vi "Text control 2 v4.9_pump-specific.vi"() -> ()   [LabVIEW 2016]
panel:
  in  "Tab Control":enum32{"Main", "Other parameters"}(tab)
  out "Line running":i32
  out "Total lines":i32
  out "Path":path=path "C:/users/rlp38/09Apr2009LTtesting/test2.txt"
  out "I vs Vg":cluster{"Y data in":dbl[], "X data in":dbl[]}[](graph)
  out "Is":dbl format="%.2e"
  out "Id":dbl format="%.2e"
  out "Ig":dbl format="%.2e"
  out "Id max vs time":cluster{"Y data in":dbl[], "X data in":dbl[]}[](graph)
  out "Id min vs time":cluster{"Y data in":dbl[], "X data in":dbl[]}[](graph)
  out "I vs Vd":cluster{"Y data in":dbl[], "X data in":dbl[]}[](graph)
  in  "Program":string="#-------------------------------------------------------\n# Liquid cycling script\n# Version 0.1\n# Author: Dimitrios Simatos\n# Last updated: 2017-10-12\n#-------------------------------------------------------\n# Things to do before running the script:\n# Set time units to minutes.\n# Set filenames.\n# Replace the tubing, if necessary.\n#-------------------------------------------------------\n# Port connections\n# Port 1: Waste\n# Port 2: Device\n# Port 3: Ultrapure water\n# Port 4: Nothing\n# Port 5: Nothing\n# Port 6: Nothing\n#-------------------------------------------------------\n# Execution time: 4 x 30 = 120 minutes = 2 hours\n# This script is designed to perform a cycling experiment between two liquids.\n# There are 4 pumping cycles, each one followed by 30 minutes of measurements.\n# All cycles pump ultrapure water (port 3).\n# Flow V = 20 pulses/second (400 ul/min)\n#-------------------------------------------------------\n# Cycle 1\npump /1ZR #initialize pump\npump /1Q #query pump\ntransfer d 1 -1 -0.1 -1 -1 0\npump /1? #report absolute plunger position\npump /1?6 #report valve position\nwait-min 1 #wait 1 minute\ntransfer d 1 -1 -0.1 -1 -1 0\npump /1N0R #set step resolution: 0.01 mm\npump /1Q #query pump\npump /1? #report absolute plunger position (the plunger should be at 0)\npump /1?6 #report valve position\nwait 1000 #wait 1 second\npump /1V300R #choose speed: 300 steps/s\npump /1Q #query pump\nwait 1000 #wait 1 second\npump /1O3R #go to port 3, counterclockwise rotation\npump /1Q #query pump\nwait 1000 #wait 1 second\npump /1A2400R #go to absolute position 2400\nwait 20000 #wait 20 seconds\npump /1V20R #set speed to 20 steps/s\npump /1Q #query pump\nwait 10000 # wait 10 seconds\ntransfer d 1 -1 -0.1 -1 -1 0\npump /1? #report absolute plunger position (the plunger should have finished moving)\npump /1?6 #report valve position\npump /1O2R #switch to port 2, counterclockwise rotation\npump /1Q #query pump\nwait 200 #wait 200 milliseconds\npump /1A0R #go to absolute position 0 (= empty syringe)\npump /1Q #query pump\npump /1? #report absolute plunger position (the plunger should be moving to 0)\npump /1?6 #report valve position\ntransfer d 1 -1 -0.1 -1 -1 0\nwait-min 1\npump /1Q #query pump\npump /1? #report absolute plunger position (the plunger should be moving to 0)\npump /1?6 #report valve position\ntransfer d 1 -1 -0.1 -1 -1 0\nwait-min 1\npump /1Q #query pump\npump /1? #report absolute plunger position\npump /1?6 #report valve position\ntransfer d 1 -1 -0.1 -1 -1 0\nwait-min 1\npump /1Q #query pump\npump /1? #report absolute plunger position\npump /1?6 #report valve position\ntransfer d 1 -1 -0.1 -1 -1 0\nwait-min 1\npump /1Q #query pump\npump /1? #report absolute plunger position\npump /1?6 #report valve position\ntransfer d 1 -1 -0.1 -1 -1 0\nwait-min 1\npump /1Q #query pump\npump /1? #report absolute plunger position\npump /1?6 #report valve position\ntransfer d 1 -1 -0.1 -1 -1 0\nwait-min 1\npump /1Q #query pump\npump /1? #report absolute plunger position\npump /1?6 #report valve position\ntransfer d 1 -1 -0.1 -1 -1 0\nwait-min 1\npump /1Q #query pump\npump /1? #report absolute plunger position\npump /1?6 #report valve position\ntransfer d 1 -1 -0.1 -1 -1 0\nwait-min 1\npump /1Q #query pump\npump /1? #report absolute plunger position\npump /1?6 #report valve position\ntransfer d 1 -1 -0.1 -1 -1 0\nwait-min 1\npump /1Q #query pump\npump /1? #report absolute plunger position\npump /1?6 #report valve position\ntransfer d 1 -1 -0.1 -1 -1 0\nwait-min 1\npump /1Q #query pump\npump /1? #report absolute plunger position\npump /1?6 #report valve position\ntransfer d 1 -1 -0.1 -1 -1 0\nwait-min 1\npump /1Q #query pump\npump /1? #report absolute plunger position\npump /1?6 #report valve position\ntransfer d 1 -1 -0.1 -1 -1 0\nwait-min 1\npump /1Q #query pump\npump /1? #report absolute plunger position\npump /1?6 #report valve position\ntransfer d 1 -1 -0.1 -1 -1 0\nwait-min 1\npump /1Q #query pump\npump /1? #report absolute plunger position\npump /1?6 #report valve position\ntransfer d 1 -1 -0.1 -1 -1 0\nwait-min 1\npump /1Q #query pump\npump /1? #report absolute plunger position\npump /1?6 #report valve position\ntransfer d 1 -1 -0.1 -1 -1 0\nwait-min 1\npump /1Q #query pump\npump /1? #report absolute plunger position\npump /1?6 #report valve position\ntransfer d 1 -1 -0.1 -1 -1 0\nwait-min 1\npump /1Q #query pump\npump /1? #report absolute plunger position\npump /1?6 #report valve position\ntransfer d 1 -1 -0.1 -1 -1 0\nwait-min 1\npump /1Q #query pump\npump /1? #report absolute plunger position\npump /1?6 #report valve position\ntransfer d 1 -1 -0.1 -1 -1 0\nwait-min 1\npump /1Q #query pump\npump /1? #report absolute plunger position\npump /1?6 #report valve position\ntransfer d 1 -1 -0.1 -1 -1 0\nwait-min 1\npump /1Q #query pump\npump /1? #report absolute plunger position\npump /1?6 #report valve position\ntransfer d 1 -1 -0.1 -1 -1 0\nwait-min 1\npump /1Q #query pump\npump /1? #report absolute plunger position\npump /1?6 #report valve position\ntransfer d 1 -1 -0.1 -1 -1 0\nwait-min 1\npump /1Q #query pump\npump /1? #report absolute plunger position\npump /1?6 #report valve position\ntransfer d 1 -1 -0.1 -1 -1 0\nwait-min 1\npump /1Q #query pump\npump /1? #report absolute plunger position\npump /1?6 #report valve position\ntransfer d 1 -1 -0.1 -1 -1 0\nwait-min 1\npump /1Q #query pump\npump /1? #report absolute plunger position\npump /1?6 #report valve position\ntransfer d 1 -1 -0.1 -1 -1 0\nwait-min 1\npump /1Q #query pump\npump /1? #report absolute plunger position\npump /1?6 #report valve position\ntransfer d 1 -1 -0.1 -1 -1 0\nwait-min 1\n#-------------------------------------------------------\n# Cycle 2\npump /1ZR #initialize pump\npump /1Q #query pump\ntransfer d 1 -1 -0.1 -1 -1 0\npump /1? #report absolute plunger position\npump /1?6 #report valve position\nwait-min 1 #wait 1 minute\ntransfer d 1 -1 -0.1 -1 -1 0\npump /1N0R #set step resolution: 0.01 mm\npump /1Q #query pump\npump /1? #report absolute plunger position (the plunger should be at 0)\npump /1?6 #report valve position\nwait 1000 #wait 1 second\npump /1V300R #choose speed: 300 steps/s\npump /1Q #query pump\nwait 1000 #wait 1 second\npump /1O3R #go to port 3, counterclockwise rotation\npump /1Q #query pump\nwait 1000 #wait 1 second\npump /1A2400R #go to absolute position 2400\nwait 20000 #wait 20 seconds\ntransfer d 1 -1 -0.1 -1 -1 0\npump /1V20R #set speed to 20 steps/s\npump /1Q #query pump\nwait 10000 # wait 10 seconds\npump /1? #report absolute plunger position (the plunger should have finished moving)\npump /1?6 #report valve position\npump /1O2R #switch to port 2, counterclockwise rotation\npump /1Q #query pump\nwait 200 #wait 200 milliseconds\npump /1A0R #go to absolute position 0 (= empty syringe)\npump /1Q #query pump\npump /1? #report absolute plunger position (the plunger should be moving to 0)\npump /1?6 #report valve position\ntransfer d 1 -1 -0.1 -1 -1 0\nwait-min 1\npump /1Q #query pump\npump /1? #report absolute plunger position (the plunger should be moving to 0)\npump /1?6 #report valve position\ntransfer d 1 -1 -0.1 -1 -1 0\nwait-min 1\npump /1Q #query pump\npump /1? #report absolute plunger position\npump /1?6 #report valve position\ntransfer d 1 -1 -0.1 -1 -1 0\nwait-min 1\npump /1Q #query pump\npump /1? #report absolute plunger position\npump /1?6 #report valve position\ntransfer d 1 -1 -0.1 -1 -1 0\nwait-min 1\npump /1Q #query pump\npump /1? #report absolute plunger position\npump /1?6 #report valve position\ntransfer d 1 -1 -0.1 -1 -1 0\nwait-min 1\npump /1Q #query pump\npump /1? #report absolute plunger position\npump /1?6 #report valve position\ntransfer d 1 -1 -0.1 -1 -1 0\nwait-min 1\npump /1Q #query pump\npump /1? #report absolute plunger position\npump /1?6 #report valve position\ntransfer d 1 -1 -0.1 -1 -1 0\nwait-min 1\npump /1Q #query pump\npump /1? #report absolute plunger position\npump /1?6 #report valve position\ntransfer d 1 -1 -0.1 -1 -1 0\nwait-min 1\npump /1Q #query pump\npump /1? #report absolute plunger position\npump /1?6 #report valve position\ntransfer d 1 -1 -0.1 -1 -1 0\nwait-min 1\npump /1Q #query pump\npump /1? #report absolute plunger position\npump /1?6 #report valve position\ntransfer d 1 -1 -0.1 -1 -1 0\nwait-min 1\npump /1Q #query pump\npump /1? #report absolute plunger position\npump /1?6 #report valve position\ntransfer d 1 -1 -0.1 -1 -1 0\nwait-min 1\npump /1Q #query pump\npump /1? #report absolute plunger position\npump /1?6 #report valve position\ntransfer d 1 -1 -0.1 -1 -1 0\nwait-min 1\npump /1Q #query pump\npump /1? #report absolute plunger position\npump /1?6 #report valve position\ntransfer d 1 -1 -0.1 -1 -1 0\nwait-min 1\npump /1Q #query pump\npump /1? #report absolute plunger position\npump /1?6 #report valve position\ntransfer d 1 -1 -0.1 -1 -1 0\nwait-min 1\npump /1Q #query pump\npump /1? #report absolute plunger position\npump /1?6 #report valve position\ntransfer d 1 -1 -0.1 -1 -1 0\nwait-min 1\npump /1Q #query pump\npump /1? #report absolute plunger position\npump /1?6 #report valve position\ntransfer d 1 -1 -0.1 -1 -1 0\nwait-min 1\npump /1Q #query pump\npump /1? #report absolute plunger position\npump /1?6 #report valve position\ntransfer d 1 -1 -0.1 -1 -1 0\nwait-min 1\npump /1Q #query pump\npump /1? #report absolute plunger position\npump /1?6 #report valve position\ntransfer d 1 -1 -0.1 -1 -1 0\nwait-min 1\npump /1Q #query pump\npump /1? #report absolute plunger position\npump /1?6 #report valve position\ntransfer d 1 -1 -0.1 -1 -1 0\nwait-min 1\npump /1Q #query pump\npump /1? #report absolute plunger position\npump /1?6 #report valve position\ntransfer d 1 -1 -0.1 -1 -1 0\nwait-min 1\npump /1Q #query pump\npump /1? #report absolute plunger position\npump /1?6 #report valve position\ntransfer d 1 -1 -0.1 -1 -1 0\nwait-min 1\npump /1Q #query pump\npump /1? #report absolute plunger position\npump /1?6 #report valve position\ntransfer d 1 -1 -0.1 -1 -1 0\nwait-min 1\npump /1Q #query pump\npump /1? #report absolute plunger position\npump /1?6 #report valve position\ntransfer d 1 -1 -0.1 -1 -1 0\nwait-min 1\npump /1Q #query pump\npump /1? #report absolute plunger position\npump /1?6 #report valve position\ntransfer d 1 -1 -0.1 -1 -1 0\nwait-min 1\npump /1Q #query pump\npump /1? #report absolute plunger position\npump /1?6 #report valve position\ntransfer d 1 -1 -0.1 -1 -1 0\nwait-min 1\n#-------------------------------------------------------\n# Cycle 3\npump /1ZR #initialize pump\npump /1Q #query pump\ntransfer d 1 -1 -0.1 -1 -1 0\npump /1? #report absolute plunger position\npump /1?6 #report valve position\nwait-min 1 #wait 1 minute\ntransfer d 1 -1 -0.1 -1 -1 0\npump /1N0R #set step resolution: 0.01 mm\npump /1Q #query pump\npump /1? #report absolute plunger position (the plunger should be at 0)\npump /1?6 #report valve position\nwait 1000 #wait 1 second\npump /1V300R #choose speed: 300 steps/s\npump /1Q #query pump\nwait 1000 #wait 1 second\npump /1O3R #go to port 3, counterclockwise rotation\npump /1Q #query pump\nwait 1000 #wait 1 second\npump /1A2400R #go to absolute position 2400\nwait 20000 #wait 20 seconds\ntransfer d 1 -1 -0.1 -1 -1 0\npump /1V20R #set speed to 20 steps/s\npump /1Q #query pump\nwait 10000 # wait 10 seconds\npump /1? #report absolute plunger position (the plunger should have finished moving)\npump /1?6 #report valve position\npump /1O2R #switch to port 2, counterclockwise rotation\npump /1Q #query pump\nwait 200 #wait 200 milliseconds\npump /1A0R #go to absolute position 0 (= empty syringe)\npump /1Q #query pump\npump /1? #report absolute plunger position (the plunger should be moving to 0)\npump /1?6 #report valve position\ntransfer d 1 -1 -0.1 -1 -1 0\nwait-min 1\npump /1Q #query pump\npump /1? #report absolute plunger position (the plunger should be moving to 0)\npump /1?6 #report valve position\ntransfer d 1 -1 -0.1 -1 -1 0\nwait-min 1\npump /1Q #query pump\npump /1? #report absolute plunger position\npump /1?6 #report valve position\ntransfer d 1 -1 -0.1 -1 -1 0\nwait-min 1\npump /1Q #query pump\npump /1? #report absolute plunger position\npump /1?6 #report valve position\ntransfer d 1 -1 -0.1 -1 -1 0\nwait-min 1\npump /1Q #query pump\npump /1? #report absolute plunger position\npump /1?6 #report valve position\ntransfer d 1 -1 -0.1 -1 -1 0\nwait-min 1\npump /1Q #query pump\npump /1? #report absolute plunger position\npump /1?6 #report valve position\ntransfer d 1 -1 -0.1 -1 -1 0\nwait-min 1\npump /1Q #query pump\npump /1? #report absolute plunger position\npump /1?6 #report valve position\ntransfer d 1 -1 -0.1 -1 -1 0\nwait-min 1\npump /1Q #query pump\npump /1? #report absolute plunger position\npump /1?6 #report valve position\ntransfer d 1 -1 -0.1 -1 -1 0\nwait-min 1\npump /1Q #query pump\npump /1? #report absolute plunger position\npump /1?6 #report valve position\ntransfer d 1 -1 -0.1 -1 -1 0\nwait-min 1\npump /1Q #query pump\npump /1? #report absolute plunger position\npump /1?6 #report valve position\ntransfer d 1 -1 -0.1 -1 -1 0\nwait-min 1\npump /1Q #query pump\npump /1? #report absolute plunger position\npump /1?6 #report valve position\ntransfer d 1 -1 -0.1 -1 -1 0\nwait-min 1\npump /1Q #query pump\npump /1? #report absolute plunger position\npump /1?6 #report valve position\ntransfer d 1 -1 -0.1 -1 -1 0\nwait-min 1\npump /1Q #query pump\npump /1? #report absolute plunger position\npump /1?6 #report valve position\ntransfer d 1 -1 -0.1 -1 -1 0\nwait-min 1\npump /1Q #query pump\npump /1? #report absolute plunger position\npump /1?6 #report valve position\ntransfer d 1 -1 -0.1 -1 -1 0\nwait-min 1\npump /1Q #query pump\npump /1? #report absolute plunger position\npump /1?6 #report valve position\ntransfer d 1 -1 -0.1 -1 -1 0\nwait-min 1\npump /1Q #query pump\npump /1? #report absolute plunger position\npump /1?6 #report valve position\ntransfer d 1 -1 -0.1 -1 -1 0\nwait-min 1\npump /1Q #query pump\npump /1? #report absolute plunger position\npump /1?6 #report valve position\ntransfer d 1 -1 -0.1 -1 -1 0\nwait-min 1\npump /1Q #query pump\npump /1? #report absolute plunger position\npump /1?6 #report valve position\ntransfer d 1 -1 -0.1 -1 -1 0\nwait-min 1\npump /1Q #query pump\npump /1? #report absolute plunger position\npump /1?6 #report valve position\ntransfer d 1 -1 -0.1 -1 -1 0\nwait-min 1\npump /1Q #query pump\npump /1? #report absolute plunger position\npump /1?6 #report valve position\ntransfer d 1 -1 -0.1 -1 -1 0\nwait-min 1\npump /1Q #query pump\npump /1? #report absolute plunger position\npump /1?6 #report valve position\ntransfer d 1 -1 -0.1 -1 -1 0\nwait-min 1\npump /1Q #query pump\npump /1? #report absolute plunger position\npump /1?6 #report valve position\ntransfer d 1 -1 -0.1 -1 -1 0\nwait-min 1\npump /1Q #query pump\npump /1? #report absolute plunger position\npump /1?6 #report valve position\ntransfer d 1 -1 -0.1 -1 -1 0\nwait-min 1\npump /1Q #query pump\npump /1? #report absolute plunger position\npump /1?6 #report valve position\ntransfer d 1 -1 -0.1 -1 -1 0\nwait-min 1\npump /1Q #query pump\npump /1? #report absolute plunger position\npump /1?6 #report valve position\ntransfer d 1 -1 -0.1 -1 -1 0\nwait-min 1\n#-------------------------------------------------------\n# Cycle 4\npump /1ZR #initialize pump\npump /1Q #query pump\ntransfer d 1 -1 -0.1 -1 -1 0\npump /1? #report absolute plunger position\npump /1?6 #report valve position\nwait-min 1 #wait 1 minute\ntransfer d 1 -1 -0.1 -1 -1 0\npump /1N0R #set step resolution: 0.01 mm\npump /1Q #query pump\npump /1? #report absolute plunger position (the plunger should be at 0)\npump /1?6 #report valve position\nwait 1000 #wait 1 second\npump /1V300R #choose speed: 300 steps/s\npump /1Q #query pump\nwait 1000 #wait 1 second\npump /1O3R #go to port 3, counterclockwise rotation\npump /1Q #query pump\nwait 1000 #wait 1 second\npump /1A2400R #go to absolute position 2400\nwait 20000 #wait 20 seconds\ntransfer d 1 -1 -0.1 -1 -1 0\npump /1V20R #set speed to 20 steps/s\npump /1Q #query pump\nwait 10000 # wait 10 seconds\npump /1? #report absolute plunger position (the plunger should have finished moving)\npump /1?6 #report valve position\npump /1O2R #switch to port 2, counterclockwise rotation\npump /1Q #query pump\nwait 200 #wait 200 milliseconds\npump /1A0R #go to absolute position 0 (= empty syringe)\npump /1Q #query pump\npump /1? #report absolute plunger position (the plunger should be moving to 0)\npump /1?6 #report valve position\ntransfer d 1 -1 -0.1 -1 -1 0\nwait-min 1\npump /1Q #query pump\npump /1? #report absolute plunger position (the plunger should be moving to 0)\npump /1?6 #report valve position\ntransfer d 1 -1 -0.1 -1 -1 0\nwait-min 1\npump /1Q #query pump\npump /1? #report absolute plunger position\npump /1?6 #report valve position\ntransfer d 1 -1 -0.1 -1 -1 0\nwait-min 1\npump /1Q #query pump\npump /1? #report absolute plunger position\npump /1?6 #report valve position\ntransfer d 1 -1 -0.1 -1 -1 0\nwait-min 1\npump /1Q #query pump\npump /1? #report absolute plunger position\npump /1?6 #report valve position\ntransfer d 1 -1 -0.1 -1 -1 0\nwait-min 1\npump /1Q #query pump\npump /1? #report absolute plunger position\npump /1?6 #report valve position\ntransfer d 1 -1 -0.1 -1 -1 0\nwait-min 1\npump /1Q #query pump\npump /1? #report absolute plunger position\npump /1?6 #report valve position\ntransfer d 1 -1 -0.1 -1 -1 0\nwait-min 1\npump /1Q #query pump\npump /1? #report absolute plunger position\npump /1?6 #report valve position\ntransfer d 1 -1 -0.1 -1 -1 0\nwait-min 1\npump /1Q #query pump\npump /1? #report absolute plunger position\npump /1?6 #report valve position\ntransfer d 1 -1 -0.1 -1 -1 0\nwait-min 1\npump /1Q #query pump\npump /1? #report absolute plunger position\npump /1?6 #report valve position\ntransfer d 1 -1 -0.1 -1 -1 0\nwait-min 1\npump /1Q #query pump\npump /1? #report absolute plunger position\npump /1?6 #report valve position\ntransfer d 1 -1 -0.1 -1 -1 0\nwait-min 1\npump /1Q #query pump\npump /1? #report absolute plunger position\npump /1?6 #report valve position\ntransfer d 1 -1 -0.1 -1 -1 0\nwait-min 1\npump /1Q #query pump\npump /1? #report absolute plunger position\npump /1?6 #report valve position\ntransfer d 1 -1 -0.1 -1 -1 0\nwait-min 1\npump /1Q #query pump\npump /1? #report absolute plunger position\npump /1?6 #report valve position\ntransfer d 1 -1 -0.1 -1 -1 0\nwait-min 1\npump /1Q #query pump\npump /1? #report absolute plunger position\npump /1?6 #report valve position\ntransfer d 1 -1 -0.1 -1 -1 0\nwait-min 1\npump /1Q #query pump\npump /1? #report absolute plunger position\npump /1?6 #report valve position\ntransfer d 1 -1 -0.1 -1 -1 0\nwait-min 1\npump /1Q #query pump\npump /1? #report absolute plunger position\npump /1?6 #report valve position\ntransfer d 1 -1 -0.1 -1 -1 0\nwait-min 1\npump /1Q #query pump\npump /1? #report absolute plunger position\npump /1?6 #report valve position\ntransfer d 1 -1 -0.1 -1 -1 0\nwait-min 1\npump /1Q #query pump\npump /1? #report absolute plunger position\npump /1?6 #report valve position\ntransfer d 1 -1 -0.1 -1 -1 0\nwait-min 1\npump /1Q #query pump\npump /1? #report absolute plunger position\npump /1?6 #report valve position\ntransfer d 1 -1 -0.1 -1 -1 0\nwait-min 1\npump /1Q #query pump\npump /1? #report absolute plunger position\npump /1?6 #report valve position\ntransfer d 1 -1 -0.1 -1 -1 0\nwait-min 1\npump /1Q #query pump\npump /1? #report absolute plunger position\npump /1?6 #report valve position\ntransfer d 1 -1 -0.1 -1 -1 0\nwait-min 1\npump /1Q #query pump\npump /1? #report absolute plunger position\npump /1?6 #report valve position\ntransfer d 1 -1 -0.1 -1 -1 0\nwait-min 1\npump /1Q #query pump\npump /1? #report absolute plunger position\npump /1?6 #report valve position\ntransfer d 1 -1 -0.1 -1 -1 0\nwait-min 1\npump /1Q #query pump\npump /1? #report absolute plunger position\npump /1?6 #report valve position\ntransfer d 1 -1 -0.1 -1 -1 0\nwait-min 1\n#-------------------------------------------------------"
  out "Command running:":string="#output s 0 0 0 -0.008 0.008 0.002"
  out "Serial port data":string
  out "Elapsed Time":dbl caption="Elapsed Time (s)"
  in  "Units":u16(ring)=1 items=["Seconds", "Minutes", "Hours"]
  in  "Time Offset":dbl caption="Set Start Time (s)"
  in  "Reset":bool
  in  "Auto Reset":bool
  in  "integration time":u32(slide) max=2 step=1 scale=0.0..2.0
  in  "Interrupt run":bool
  out "Absolute plunger position vs time":cluster{"Y data in":dbl[], "X data in":dbl[]}[](graph)
  out "Valve position vs time":cluster{"Y data in":dbl[], "X data in":dbl[]}[](graph)
  in  "Halt pump":bool
  in  "Hard stop pump":bool
  in  "Gate Range\nmode":u16(ring) items=["Auto", "Limited", "Fixed"]
  in  "Gate Range":u8(slide)=6 max=11 scale=0.0..11.0
  in  "Source/Drain\nRange mode":u16(ring) items=["Auto", "Limited", "Fixed"]
  in  "Source/Drain Range":u8(slide)=6 max=11 scale=0.0..11.0
  in  "Panel Controls":T1={"Emergency Stop"=refnum, "TransGraph Max"=1e-05, "Text/Graph (text=false)"=TRUE} {"TransGraph Max" format="%.2e"}
  in  "Panel Controls 2":T2={"Emergency Stop"=refnum, "TransGraph Max"=1e-05, "Text/Graph (text=false)"=TRUE, "TransGraph Min"=1e-11} {"TransGraph Min" format="%.2e"; "TransGraph Max" format="%.2e"}
  in  "SMU4":cluster{"on/off":bool, "Voltage":dbl} {"Voltage" min=-100.0 max=100.0 format="%.2f"}
  in  "Full Reset":bool
  in  "Standby":T3
  out "error out":errorcluster
  in  "Delay before read (ms)":u32=1000
  in  "byte count":u32=64
  in  "Serial End Mode for Reads":u16(ring)=2 items=["None", "LastBit", "TermChar"]
  in  "Timeout (ms)":u32=10000
  in  "Enable Termination\nChar (T)":bool=TRUE
  in  "Termination char\n(0xA = '\\n' = LF)\n(0xD = '\\r' = CR)":u8=13 format="%.0x"
  in  "flow control":u16(ring) items=["None"=0, "XON/XOFF"=1, "RTS/CTS"=2, "DTR/DSR"=4]
  in  "stop bits":u16(ring)=10 items=["1.0"=10, "1.5"=15, "2.0"=20]
  in  "parity":u16(ring) items=["None", "Odd", "Even", "Mark", "Space"]
  in  "data bits":u16=8 min=5 max=8 step=1
  in  "VISA resource name":refnum<visa-resource-name>="COM6"
  in  "baud rate":u32=9600
  in  "Drain: Compliance":dbl=0.001 format="%.8f"
  in  "Gate: Compliance":dbl=0.001 format="%.8f"
  in  "hold time /s":dbl format="%.2f"
  in  "delay time /s":dbl format="%.2f"
  in  "Integration time (short)":dbl=0.0019 min=8e-05 max=0.0019 step=8e-05 format="%^.0e"
  in  "Integration time (long)":dbl=0.32 min=0.04 max=2.0 step=0.02 format="%.2f"
  in  "Step delay /s":dbl format="%.2f"
  in  "Prefix (transfer)":string="_step_1_ultrapure_H2O_"
  in  "Suffix (transfer)":string="_T.txt"
  in  "Prefix (Idmax-Idmin)":string="_step_1_ultrapure_H2O_Idmax_Idmin_vs_time_Vg=-1.0V_Vd=-1.0V"
  in  "Suffix (Idmax-Idmin)":string=".txt"
  in  "Prefix (output)":string="_step_1_ultrapure_H2O_"
  in  "Suffix (output)":string="_O.txt"
  in  "Prefix (script)":string="_step_1_ultrapure_H2O_script"
  in  "Prefix (serial port log)":string="_step_1_ultrapure_H2O_serial port output"
  in  "Prefix (plunger)":string="_step_1_ultrapure_H2O_plunger_vs_time"
  in  "Suffix (plunger)":string=".txt"
  in  "Prefix (valve)":string="_step_1_ultrapure_H2O_valve_vs_time"
  in  "Suffix (valve)":string=".txt"
  in  "Gate":T4={"Gate Start"=0.0, "Gate Stop"=2.0, "Gate Step (linear only)"=1.0, "Gate Compliance"=0.0001, "Gate PComp"=0.0, "Range mode"=0, "Range"=6} {"Range" max=11 scale=0.0..11.0; "Range mode" items=["Auto", "Limited", "Fixed"]; "Gate PComp" format="%^.2e"; "Gate Compliance" format="%^.2e"; "Gate Step (linear only)" format="%^.4e"; "Gate Stop" format="%^.4e"; "Gate Start" format="%^.4e"}
  in  "Drain 2":T5={"Drain Start"=0.0, "Drain Stop"=2.0, "Drain Compliance"=0.0001, "Drain Step"=1.0, "Drain PComp"=0.0, "Range mode"=0, "Range"=6} {"Range" max=11 scale=0.0..11.0; "Range mode" items=["Auto", "Limited", "Fixed"]; "Drain PComp" format="%^.2e"; "Drain Step" format="%^.4e"; "Drain Compliance" format="%^.2e"; "Drain Stop" format="%^.4e"; "Drain Start" format="%^.4e"}
  in  "Timings 2":T6={"integration time"=0, "Short/Long integration time"=0.00064, "hold time (sec)"=0.0, "delay time (sec)"=0.0, "Step Time (0 disables)"=0.0, "sweep method"=0, "Pulse period"=0.005, "Base voltage"=0.0, "Pulse width"=0.0005} {"Pulse width" min=0.0005 max=0.1 step=0.0001 format="%.4f"; "Base voltage" format="%^.4e"; "Pulse period" min=0.005 max=1.0 step=0.0001 format="%.4f"; "sweep method" items=["Continuous", "Pulsed"]; "Step Time (0 disables)" format="%.2f"; "delay time (sec)" format="%.4f"; "hold time (sec)" format="%.4f"; "Short/Long integration time" format="%^.0e"; "integration time" scale=0.0..2.0}
  # "Syntax:\nitime [s|m|l]\ngaterangemode [a|l|f]\ndrainrangemode [a|l|f]\npulsed [on|off] PulsePeriod(sec) PulseBaseVoltage PulseONWidth(sec)\nstandby [on l off]\nwait NumMilliseconds\nwait-min NumMinutes\n# texthere = comment\ntransfer [s|d] VgStart VgStop VgStep VdStart VdStop VdStep\noutput [s|d] VgStart VgStop VgStep VdStart VdStop VdStep\nsample Vg Vd NumSamples Time(s) SampleInterval(s)\nsamplei Idg NumSamples Time(s) SampleInterval(s) VDGcompliance\n100 samples is approximately 13 seconds with medium integration\n# if in doubt use SampleInterval(s) = 0.004\nstressV VG VD IGcompliance IDcompliance Duration(sec)\nstressI IDG VDGcompliance Duration(sec)\nvsu2pulse Bias Duration(s)\npulsedstressV [s|d] VEstop VgON VgOFF Period(s) PulseONwidth(s) Vd\nsample-fpp Vg Vd NumSamples Time\nresample-fpp Vg Vd\ntransfer-fpp [s|d] VgStart VgStop VgStep VdStart VdStop VdStep\noutput-fpp [s|d] VgStart VgStop VgStep VdStart VdStop VdStep\nserial SerialPortCommand\npump SerialPortCommand for the OEM pump\n\nSPM OEM Pump Syntax (<x>: pump number, use 1 if only one pump):\nif the command syntax contains [R], then append the letter R to the command\n/<x>Q: query (a query command should follow each command)\n/<x>Z[R] or /<x>Y[R]: initialize pump\n/<x>N<n>[R] (<n>=0,1): <0> (<1>) microstep 0.01 mm (0.00125 mm) resolution\n/<x>I<n> (<n>=0-6): turn to port number n (clockwise)\n/<x>O<n> (<n>=0-6): turn to port number n (counterclockwise)\n/<x>X: Re-execute last command string\n/<x>G<n>[R] (<n>=0-60000): repeat command sequence (default: 0, 0=loop forever)\n/<x>g: Mark the start of a repeat sequence (max = 10)\n/<x>M<n>[R] (<n>=0-86400000): delay command execution by n milliseconds\n/<x>H: Halt; Pause the sequence after finishing the current move\n/<x>T: Hardstop; Interrupt the current move and suppress it from the sequence\n/<x>A<n>[R] (<n>=0-3000 with N=0, 0-24000 with N=1): absolute position\n/<x>P<n>[R] (<n>=0-3000 with N=0, 0-24000 with N=1): relative pickup\n/<x>D<n>[R] (<n>=0-3000 with N=0, 0-24000 with N=1): relative dispense\n/<x>V<n>[R] (<n>=5-1600 default: 150): set peak speed (pulses/sec)\n/<x>S<n>[R] (<n>=10-40 default: 22): set speed (NOT in pulses/sec, look in manual)\nNOTE: When controlled with absolute position, one does not need to pay special attention to the syringe that is mounted on the pump.\nWithdraw from lower stage (ports 3, 5), dispense from higher stage (ports 2, 4, 6).\nConnect Port 1 to waste."
  # "Time"
  # "1\n2\n3\n4\n5\n6\n7\n8\n9\n10\n11\n12\n13\n14\n15\n16\n17\n18\n19\n20"
  # "Serial port settings"
  # "Filename settings"
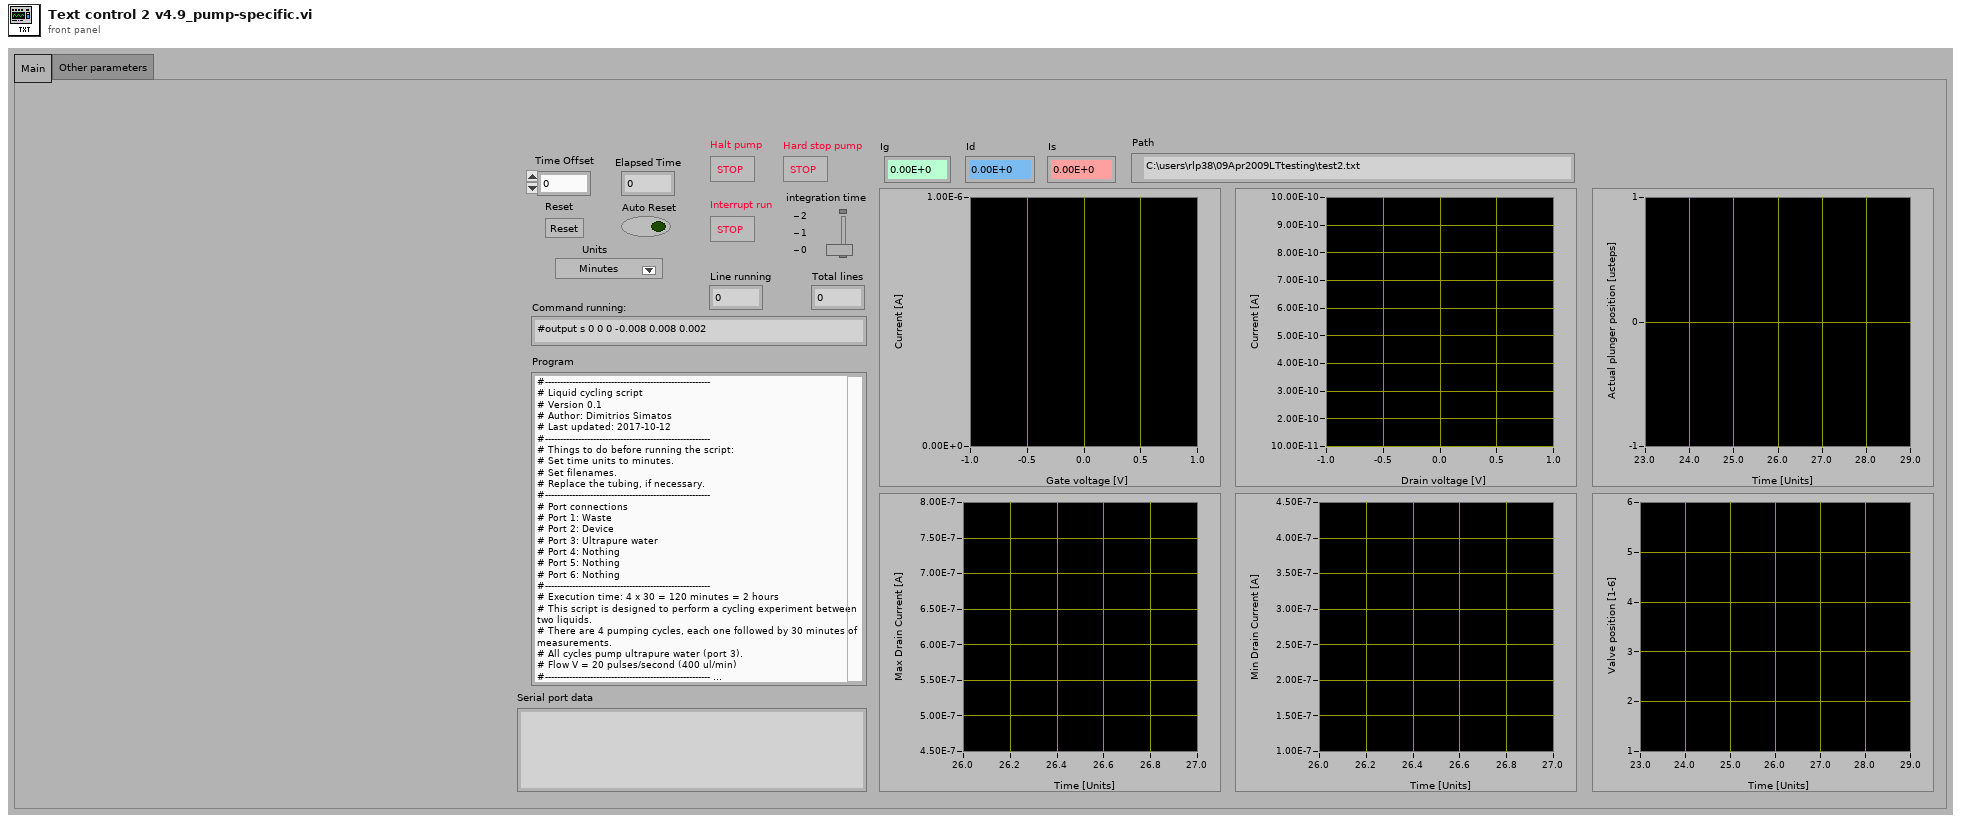
[diagram p1: front panel]
types:
  T1 = cluster{"Emergency Stop":refnum<vi>, "TransGraph Max":dbl, "Text/Graph (text=false)":bool}
  T2 = cluster{"Emergency Stop":refnum<vi>, "TransGraph Max":dbl, "Text/Graph (text=false)":bool, "TransGraph Min":dbl}
  T3 = cluster{"Gate Standby":bool, "Drain Standby":bool}
  T4 = cluster{"Gate Start":dbl, "Gate Stop":dbl, "Gate Step (linear only)":dbl, "Gate Compliance":dbl, "Gate PComp":dbl, "Range mode":u16, "Range":u8}
  T5 = cluster{"Drain Start":dbl, "Drain Stop":dbl, "Drain Compliance":dbl, "Drain Step":dbl, "Drain PComp":dbl, "Range mode":u16, "Range":u8}
  T6 = cluster{"integration time":u32, "Short/Long integration time":dbl, "hold time (sec)":dbl, "delay time (sec)":dbl, "Step Time (0 disables)":dbl, "sweep method":u16, "Pulse period":dbl, "Base voltage":dbl, "Pulse width":dbl}
  T7 = enum16{"open", "replace", "create", "open or create", "replace or create", "replace or create with confirmation"}
  T8 = cluster{"V2 Start":dbl, "V2 Step":dbl, "Number of points":i32}
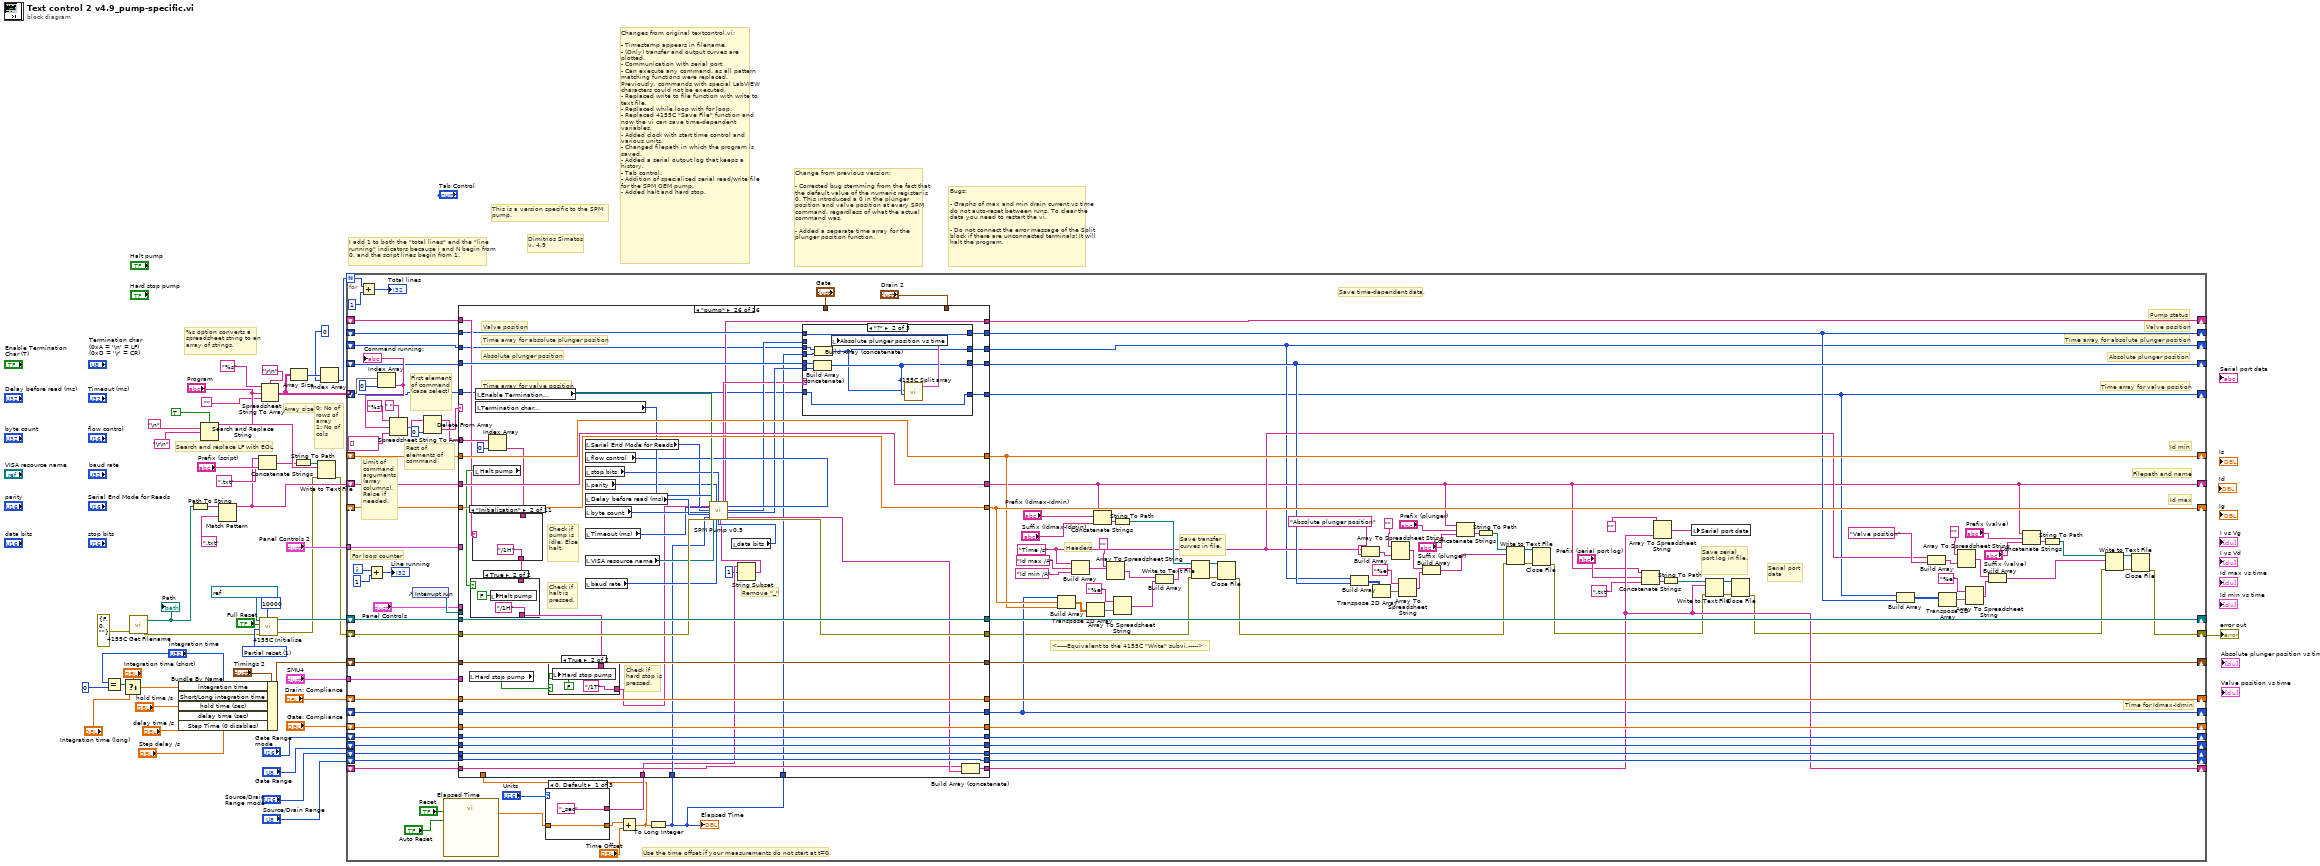
[diagram p0: block diagram]
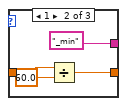
[diagram p2: hidden frame]
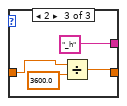
[diagram p3: hidden frame]
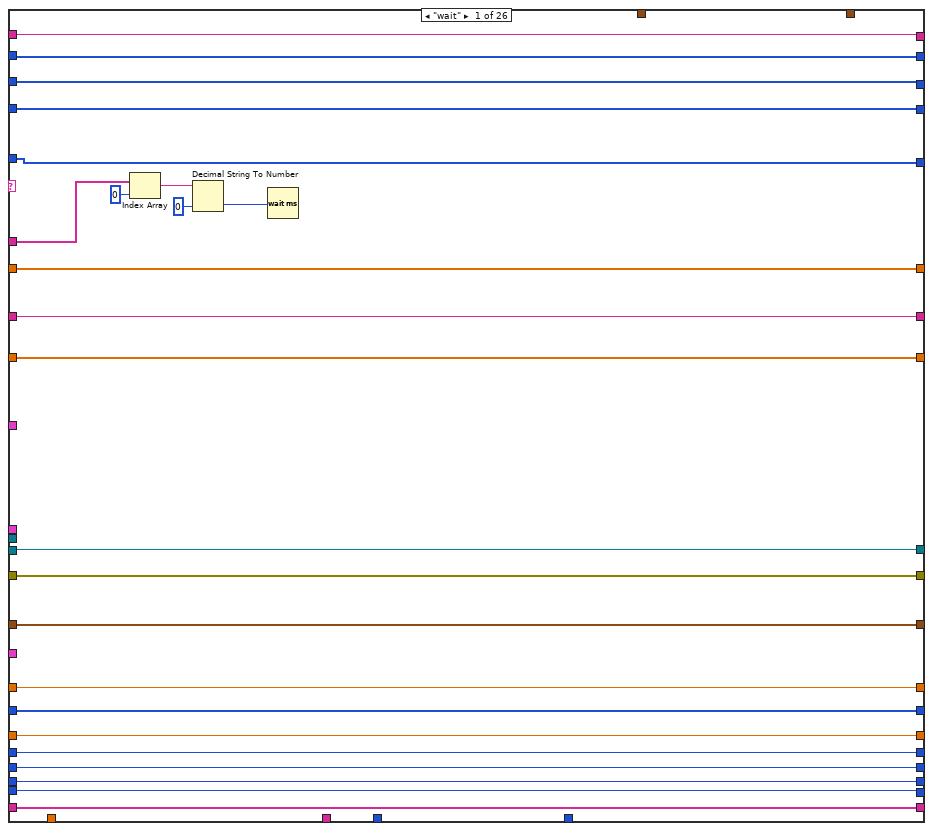
[diagram p4: hidden frame]
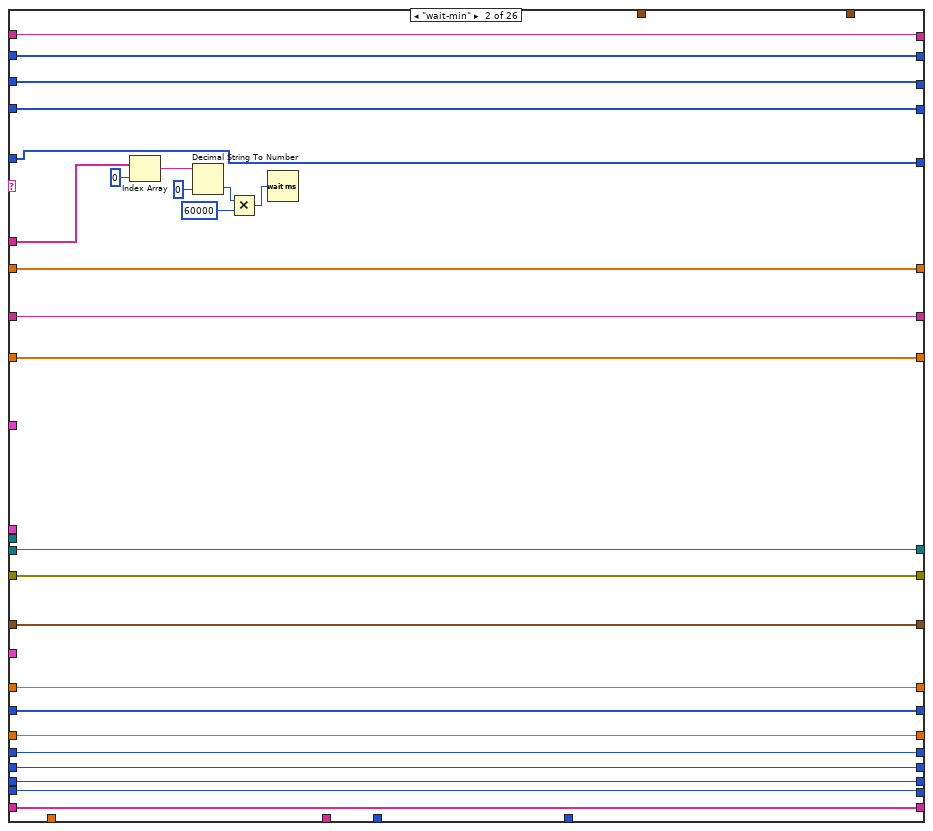
[diagram p5: hidden frame]
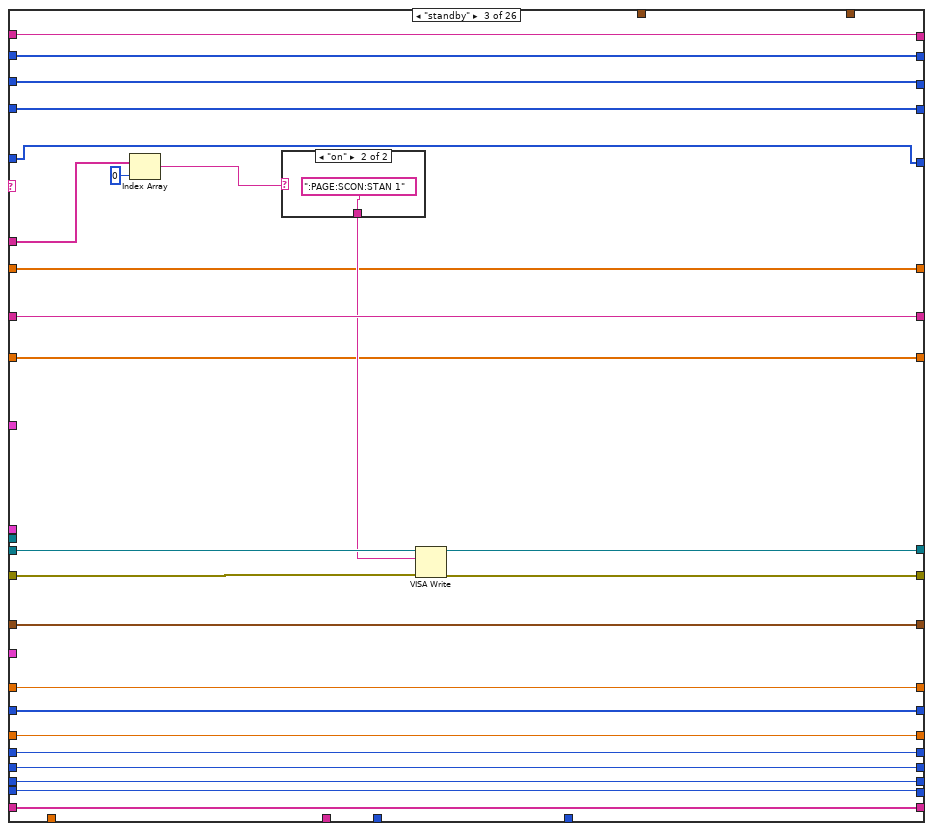
[diagram p6: hidden frame]
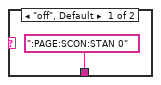
[diagram p7: hidden frame]
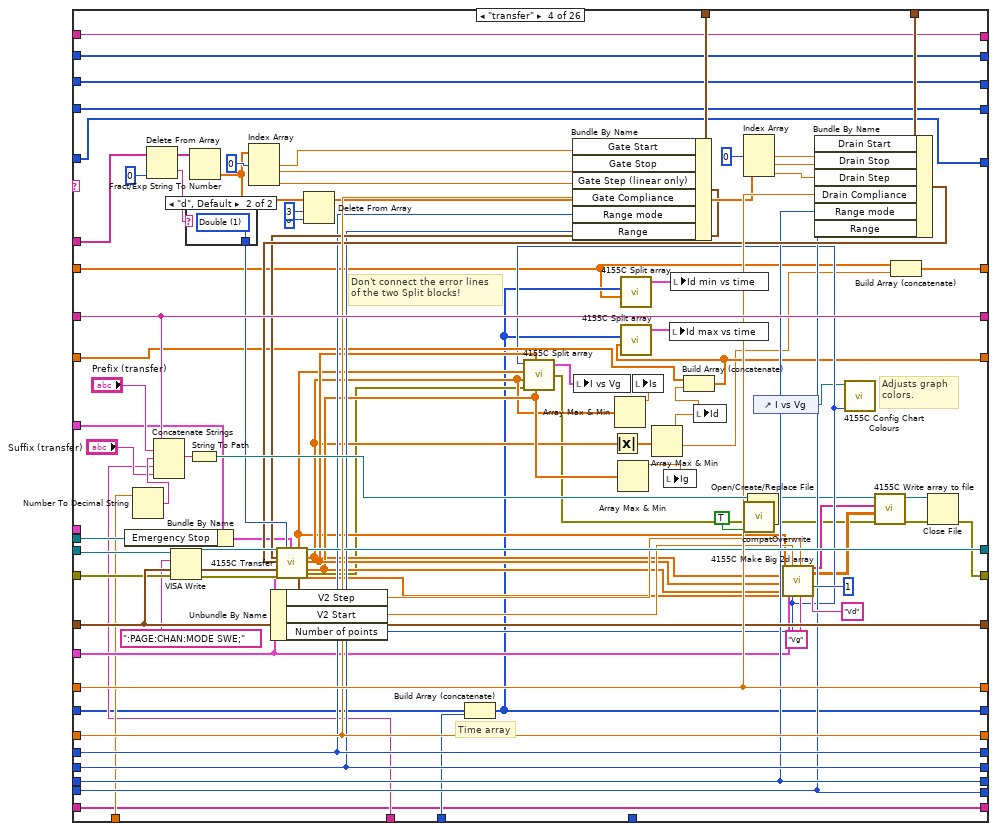
[diagram p8: hidden frame]
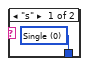
[diagram p9: hidden frame]
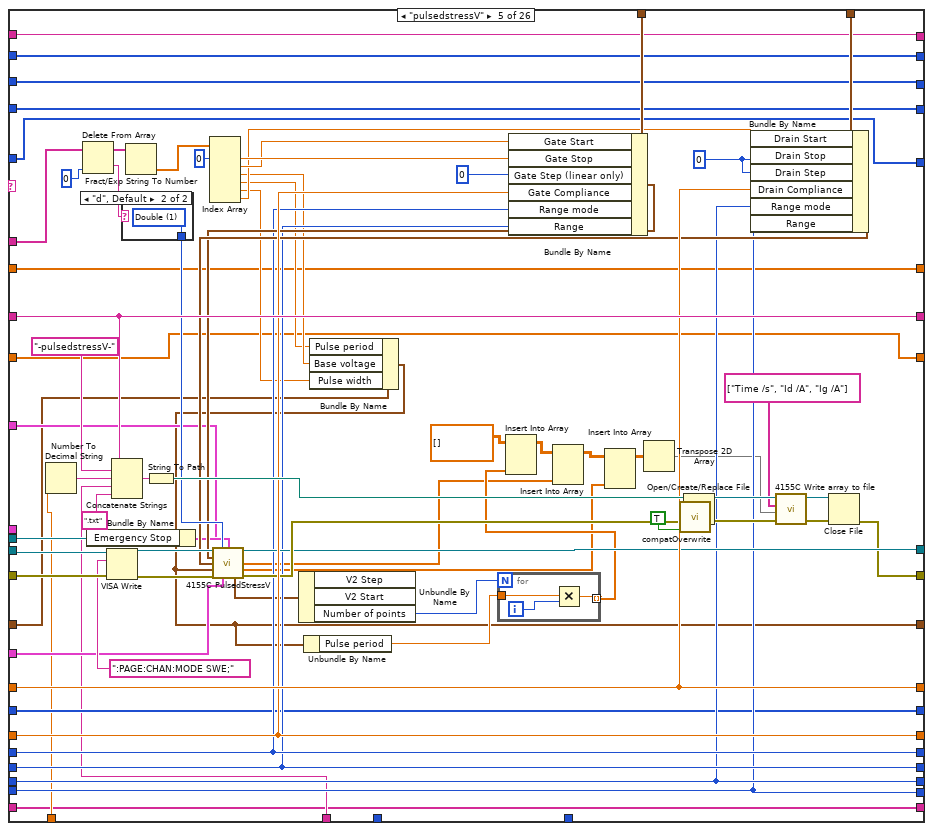
[diagram p10: hidden frame]
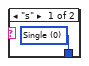
[diagram p11: hidden frame]
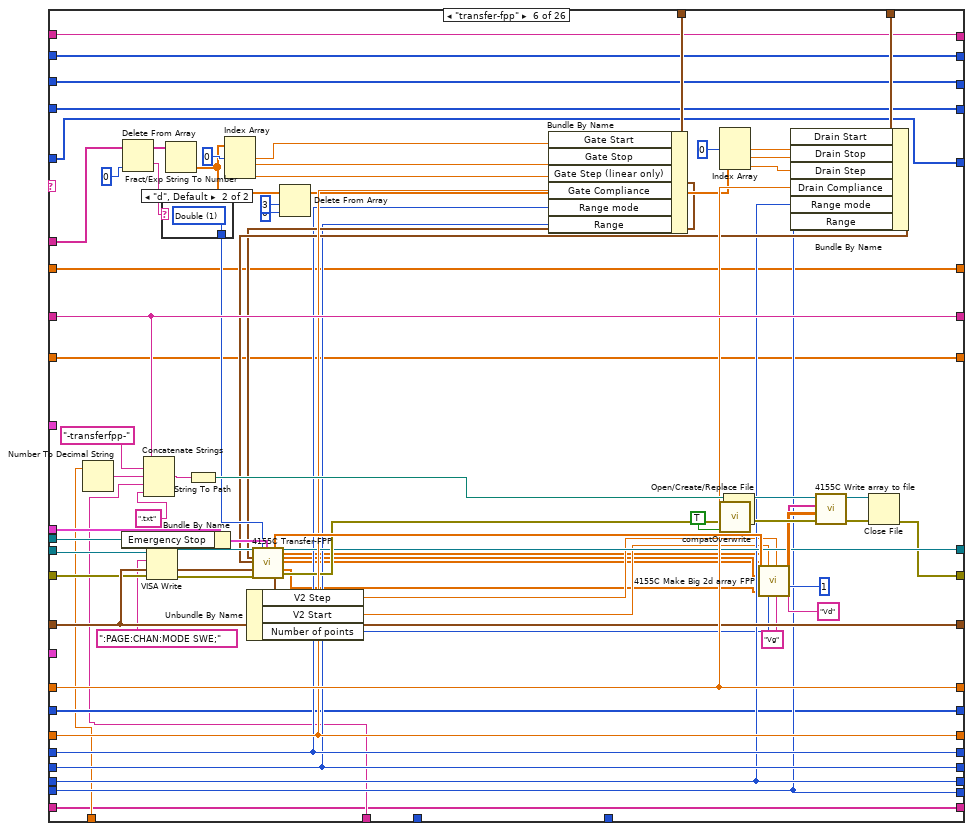
[diagram p12: hidden frame]
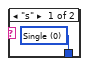
[diagram p13: hidden frame]
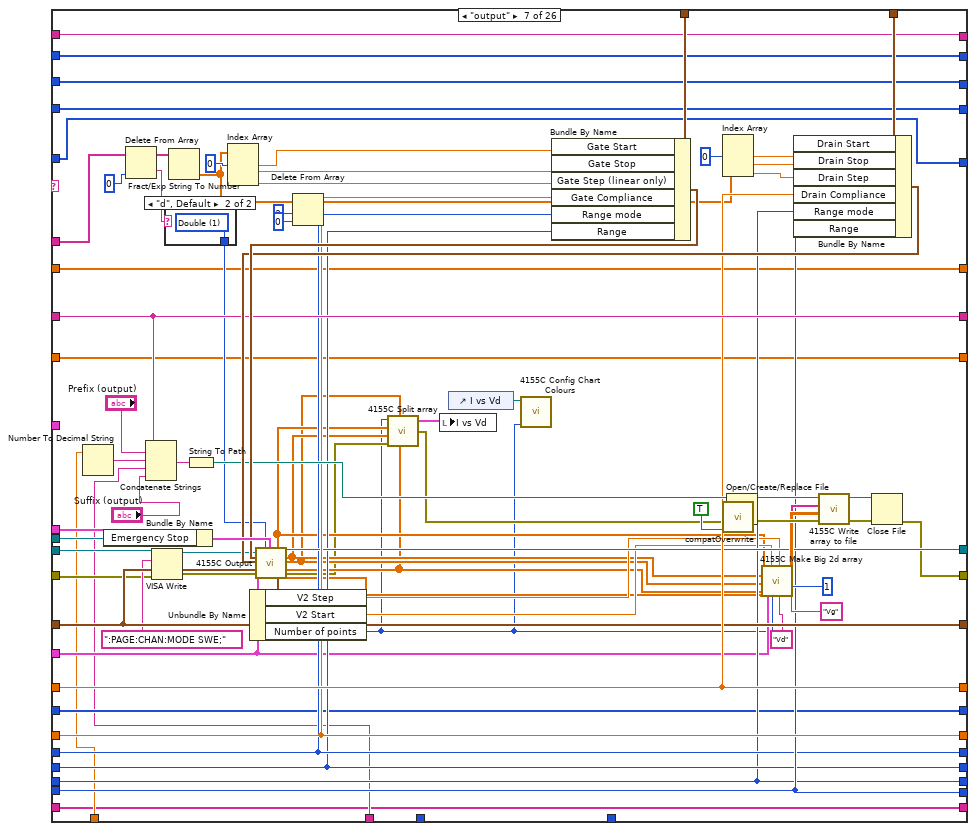
[diagram p14: hidden frame]
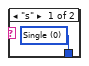
[diagram p15: hidden frame]
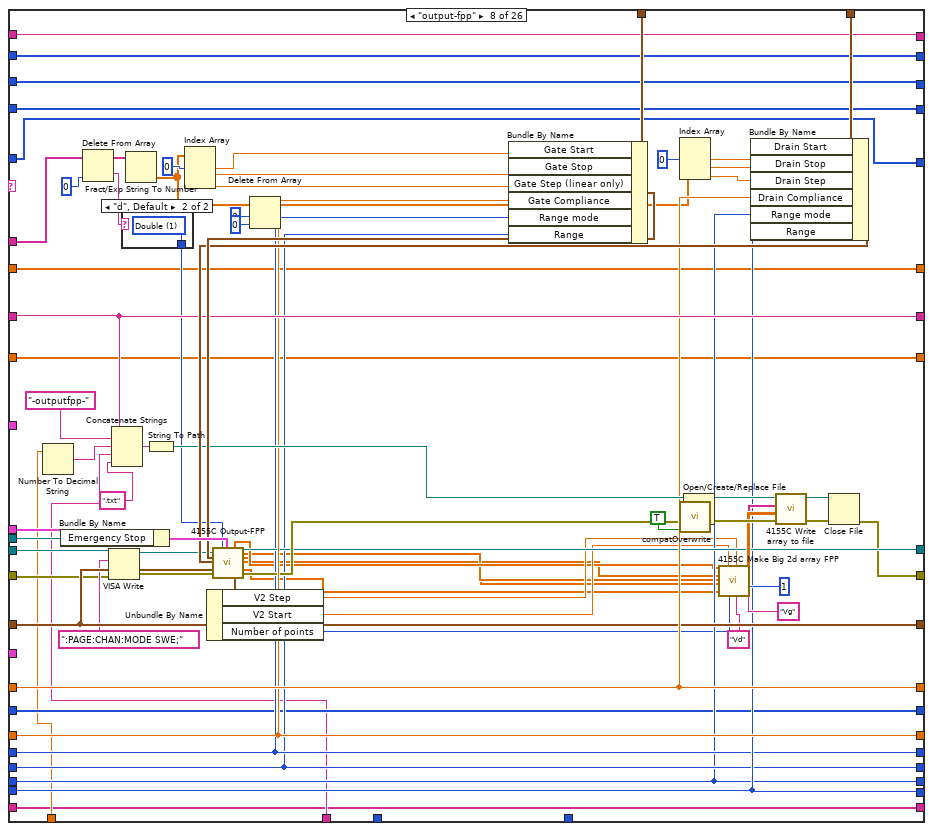
[diagram p16: hidden frame]
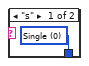
[diagram p17: hidden frame]
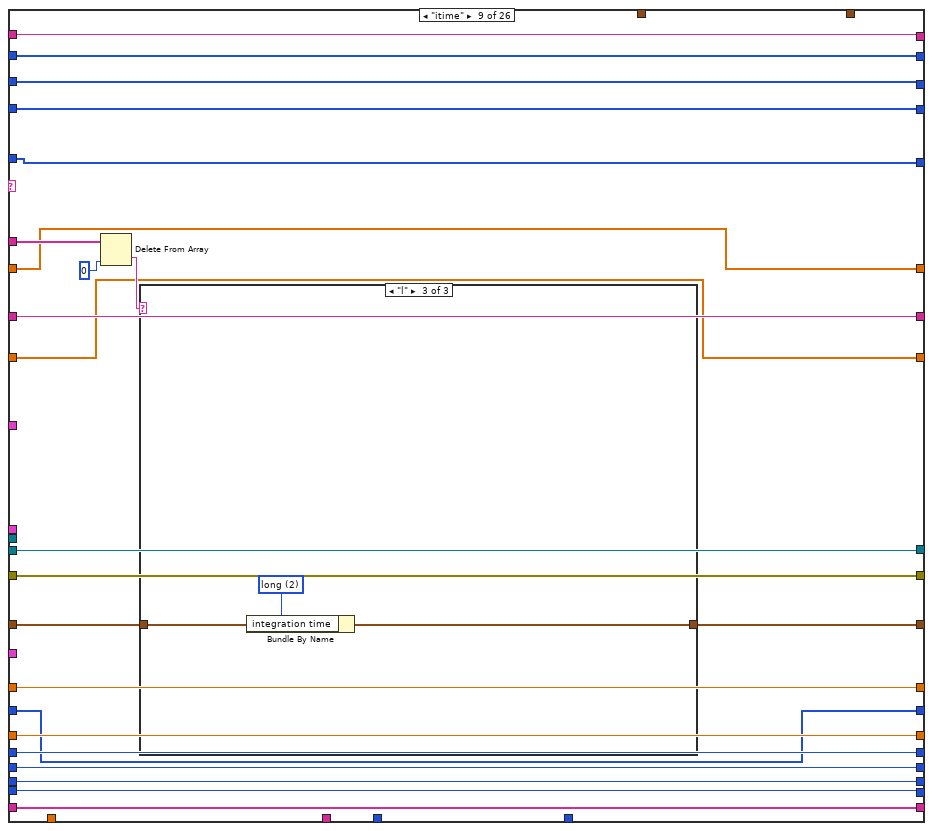
[diagram p18: hidden frame]
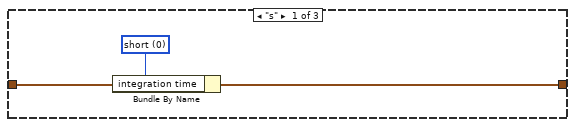
[diagram p19: hidden frame]
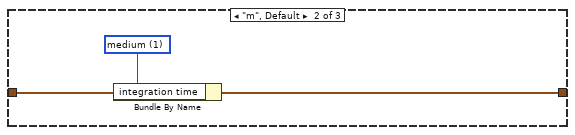
[diagram p20: hidden frame]
diagram:
  w40 = u16 1 items=["Reset All", "Partial reset"] ("Type of reset")
  # "Change from previous version:\n\n- Corrected bug stemming from the fact that the default value of the numeric register is 0. This introduced a 0 in the plunger position and valve position at every SPM command, regardless of what the actual command was.\n\n- Added a separate time array for the plunger position function."
  # "This is a version specific to the SPM pump."
  # "I add 1 to both the \"total lines\" and the \"line running\" indicators because i and N begin from 0, and the script lines begin from 1."
  # "Bugs:\n\n- Graphs of max and min drain current vs time do not auto-reset between runs. To clear the data you need to restart the vi.\n\n- Do not connect the error message of the Split block if there are unconnected terminals! It will halt the program."
  # "Array size"
  # "%s option converts a spreadsheet string to an array of strings."
  # "0: No of rows of array\n1: No of cols"
  # "Dimitrios Simatos\nv. 4.9"
  # "Changes from original textcontrol.vi:\n\n- Timestamp appears in filename.\n- (Only) transfer and output curves are plotted.\n- Communication with serial port.\n- Can execute any command, as all pattern matching functions were replaced. Previously, commands with special LabVIEW characters could not be executed.\n- Replaced write to file function with write to text file.\n- Replaced while loop with for loop.\n- Replaced 4155C \"Save File\" function and now the vi can save time-dependent variables.\n- Added clock with start time control and various units.\n- Changed filepath in which the program is saved.\n- Added a serial output log that keeps a history.\n- Tab control.\n- Addition of specialized serial read/write file for the SPM OEM pump.\n- Added halt and hard stop."
  # "Search and replace LF with EOL"
  n1 = Equal?(x="integration time", y=u32 0) -> (x = y?=w44:bool)
  n2 = Select(t="Integration time (short)", s=w44, f="Integration time (long)") -> (s? t:f=w48:dbl)
  n3 = call "4155C Get Filename.vi"("error in (no error)"=errorcluster {"status"=FALSE, "code"=0, "source"=""}) -> ("error out"=w35:errorcluster, "path"=w10:path)  [unwired: 2 in, 1 out]
  "Path" <- w10
  n4 = Bundle By Name(cluster="Timings 2", "integration time"="integration time", "Short/Long integration time"=w48, "hold time (sec)"="hold time /s", "delay time (sec)"="delay time /s", "Step Time (0 disables)"="Step delay /s") -> (w33:T6)
  n5 = Path To String(path=w10) -> (string=w11:string)
  n6 = Search and Replace String(replace all?=TRUE ("replace all? (F)"), input string="Program", search string="\n", replace string="\r\n") -> (result string=w23:string)  [unwired: 4 in, 3 out]
  n7 = Match Pattern(string=w11, regular expression=".txt") -> (before substring=w5:string)  [unwired: 1 in, 3 out]
  n8 = Concatenate Strings(w5, "Prefix (script)", ".txt" ("regular expression")) -> (w4:string)
  n9 = call "4155C Initialise.vi"("VISA resource name in"=refnum<visa-resource-name> "GPIB0::14::INSTR", "Reset"="Full Reset", "Type of reset"=w40, "error in (no error)"=w35, "VISA Timeout Value"=u32 10000) -> ("VISA Resource Name out"=w34:refnum<visa-resource-name>, "error out"=w2:errorcluster)
  n10 = Spreadsheet String To Array(delimiter (Tab)="\r\n", format string="%s", spreadsheet string="Program", array type (2D Dbl)="") -> (array=w14:string[][])
  n11 = Array Size(array=w14) -> (size(s)=w18:i32[])
  n12 = String To Path(string=w4) -> (path=w3:path)
  n13 = Write to Text File(file (use dialog)=w3, text=w23, error in=w2) -> (error out=w1:errorcluster)  [unwired: 1 in, 2 out]
  n14 = Index Array(array=w18, index=0) -> (element=w16:i32)
  n15 = for {
    N: w16 -> [w114]
    tunnel: "SMU4" -> [w155]
    shift-left: "Source/Drain Range" -> [w160]
    shift-right: [w156] -> _
    shift-left: "Source/Drain\nRange mode" -> [w161]
    shift-right: [w157] -> _
    shift-left: "Gate Range" -> [w162]
    shift-right: [w158] -> _
    shift-left: "Gate Range\nmode" -> [w163]
    shift-right: [w159] -> _
    shift-left: "Gate: Compliance" -> [w172]
    shift-right: [w168] -> _
    shift-left: "Drain: Compliance" -> [w173]
    shift-right: [w169] -> _
    shift-left: w33 -> [w174]
    shift-right: [w170] -> _
    shift-left: w1 -> [w175]
    shift-right: [w52] -> w9
    shift-left: w34 -> [w176]
    shift-right: [w171] -> _
    shift-left: w5 -> [w177]
    shift-right: [w56] -> _
    tunnel: "Panel Controls 2" -> [w154]
    shift-right: [w125] -> _
    shift-left: _ -> [w153]
    shift-right: [w79] -> _
    shift-left: _ -> [w149]
    tunnel: w14 -> [w148] mode=indexing
    shift-right: [w120] -> _
    shift-left: _ -> [w121]
    shift-right: [w103] -> _
    shift-left: _ -> [w106]
    shift-right: [w80] -> _
    shift-left: _ -> [w98]
    shift-right: [w58] -> _
    shift-left: _ -> [w97]
    shift-right: [w96] -> _
    shift-left: _ -> [w95]
    shift-right: [w51] -> _
    shift-left: _ -> [w76]
    shift-right: [w50] -> _
    shift-left: _ -> [w57]
    i -> [w109]
    w59 = "Time /s" ("element")
    # "Time array for valve position"
    # "Time array for absolute plunger position"
    # "Valve position"
    # "Pump status"
    # "Absolute plunger position"
    # "Serial port data"
    # "Save serial port log in file."
    # "For loop counter"
    # "<-----Equivalent to the 4155C \"Write\" subvi.----->"
    # "Headers"
    # "Save transfer curves in file."
    # "Filepath and name"
    # "Save time-dependent data."
    # "Use the time offset if your measurements do not start at t=0."
    # "Time for Idmax-Idmin"
    # "Rest of elements of command"
    # "Id min"
    # "Id max"
    # "Limit of command arguments (array columns). Raise if needed."
    # "First element of command\n(case select)"
    n16 = Add(x=w114, y=1) -> (x+y=→"Total lines":i32)
    n17 = Add(x=w109, y=1) -> (x+y=→"Line running":i32)
    n18 = Index Array(array=w148, index=0 ("line index")) -> (element=w143:string)
    "Command running:" <- w143
    n19 = Spreadsheet String To Array(delimiter (Tab)=" ", format string="%s", spreadsheet string=w143, array type (2D Dbl)=string[] []) -> (array=w140:string[])
    n20 = control-ref of="Interrupt run"() -> (w167:refnum<vi>)
    n21 = Delete From Array(array=w140, index=0) -> (deleted portion=w141:string, array with subset deleted=w139:string[])  [unwired: 1 in]
    n22 = call "Elapsed Time"("Reset"="Reset", "Auto Reset"="Auto Reset") -> ("Elapsed Time (s)"=w150:dbl)  [unwired: 10 in, 7 out]
    n23 = case shown="0, Default" "Units" {
      tunnel: ["_sec" "_min" "_h"] -> w151
      tunnel: [w178 w182 w185] -> w116
      tunnel: w150 -> [w178 w181 w186]
      frame 0, Default {
      }
      frame 1 {
        n24 = Divide(x=w181, y=60.0) -> (x/y=w182:dbl)
      }
      frame 2 {
        n25 = Divide(x=w186, y=3600.0) -> (x/y=w185:dbl)
      }
    }
    n26 = Add(x=w116, y="Time Offset") -> (x+y=w115:dbl)
    n27 = To Long Integer(number=w115) -> (32bit integer=w77:i32)
    "Elapsed Time" <- w77
    n28 = case shown="\"pump\"" w141 {
      tunnel: w139 -> [w211 w237 w262 w344 w415 w491 w573 w650 w695 w728 w762 w794 w822 w843 _ _ w968 w1036 _ w1115 w1166 w1215 w1292 w1361 w1388 w1444]
      tunnel: w177 -> [w206 w233 w260 w351 w422 w499 w580 w658 w684 w717 w754 w787 w816 w836 w862 w911 w946 w1018 w1056 w1102 w1153 w1203 w1286 w1357 w1390 w1446]
      tunnel: w176 -> [w205 w232 w251 w322 w406 w468 w549 w626 w685 w718 w755 w788 w817 w837 w867 w913 w974 w1042 w1060 w1121 w1172 w1221 w1298 w1315 w1394 w1450]
      tunnel: w175 -> [w204 w231 w250 w321 w405 w467 w546 w623 w686 w719 w756 w789 w818 w838 w866 w884 w973 w1041 w1059 w1120 w1171 w1220 w1297 w1314 w1393 w1449]
      tunnel: w174 -> [w203 w230 w259 w347 w381 w495 w576 w654 w694 w727 w753 w786 w815 w835 w865 w908 w937 w1010 w1065 w1095 w1146 w1196 w1285 w1356 w1395 w1451]
      tunnel: w173 -> [w202 w229 w258 w349 w420 w497 w578 w656 w693 w726 w761 w793 w821 w842 w864 w893 w972 w1040 w1068 w1119 w1170 w1219 w1296 w1365 w1396 w1452]
      tunnel: w172 -> [w201 w228 w257 w348 w419 w496 w577 w655 w692 w725 w760 w792 w820 w841 w863 w894 w947 w1019 w1067 w1103 w1154 w1204 w1287 w1358 w1398 w1453]
      tunnel: [w205 w232 w249 w346 w417 w493 w575 w652 w685 w718 w755 w788 w817 w837 w867 w913 w938 w992 w1058 w1096 w1147 w1197 w1238 w1317 w1394 w1450] -> w171
      tunnel: [w204 w231 w248 w345 w416 w492 w574 w651 w686 w719 w756 w789 w818 w838 w866 w883 w948 w993 w1057 w1104 w1155 w1205 w1237 w1316 w1392 w1448] -> w75
      tunnel: [w203 w230 w259 w347 w377 w495 w576 w654 w687 w720 w753 w786 w815 w835 w865 w908 w937 w1010 w1065 w1095 w1146 w1196 w1285 w1356 w1395 w1451] -> w170
      tunnel: [w202 w229 w258 w349 w420 w497 w578 w656 w693 w726 w761 w793 w821 w842 w864 w893 w972 w1040 w1068 w1119 w1170 w1219 w1296 w1365 w1396 w1452] -> w169
      tunnel: [w201 w228 w257 w348 w419 w496 w577 w655 w692 w725 w760 w792 w820 w841 w863 w894 w947 w1019 w1067 w1103 w1154 w1204 w1287 w1358 w1398 w1453] -> w168
      tunnel: [w206 w233 w260 w351 w422 w499 w580 w658 w684 w717 w754 w787 w816 w836 w862 w911 w946 w1018 w1056 w1102 w1153 w1203 w1286 w1357 w1390 w1446] -> w56
      tunnel: w167 -> [_ _ _ w354 w426 w504 w584 w662 _ _ _ _ _ _ _ _ w943 w1015 _ w1101 w1152 w1202 w1258 w1333 _ _]
      tunnel: "Gate" -> [_ _ _ w331 w409 w478 w560 w637 _ _ _ _ _ _ _ _ _ _ _ _ _ _ _ _ _ _]
      tunnel: "Drain 2" -> [_ _ _ w330 w408 w477 w559 w636 _ _ _ _ _ _ _ _ _ _ _ _ _ _ _ _ _ _]
      tunnel: "Panel Controls" -> [_ _ _ _ _ w476 w558 w635 _ _ _ _ _ _ _ _ _ _ _ _ _ _ _ _ _ _]
      tunnel: w163 -> [w200 w227 w256 w315 w399 w461 w544 w621 w691 w724 _ w785 w814 w834 w861 w895 w933 w1006 w1061 w1091 w1142 w1192 w1281 w1352 w1399 w1454]
      tunnel: w162 -> [w199 w226 w255 w314 w398 w460 w543 w620 w690 w723 w759 _ w805 w840 w860 w896 w934 w1007 w1062 w1092 w1143 w1193 w1282 w1353 w1400 w1455]
      tunnel: w161 -> [w198 w225 w254 w313 w397 w459 w542 w619 w689 w722 w758 w791 w819 _ w859 w897 w935 w1008 w1063 w1093 w1144 w1194 w1283 w1354 w1401 w1456]
      tunnel: w160 -> [w197 w224 w253 w312 w396 w458 w545 w622 w688 w721 w757 w790 _ w839 w858 w898 w936 w1009 w1064 w1094 w1145 w1195 w1284 w1355 w1402 w1457]
      tunnel: [w200 w227 w256 w315 w399 w461 w544 w621 w691 w724 w752 w785 w814 w834 w861 w895 w933 w1006 w1061 w1091 w1142 w1192 w1281 w1352 w1399 w1454] -> w159
      tunnel: [w199 w226 w255 w314 w398 w460 w543 w620 w690 w723 w759 w777 w805 w840 w860 w896 w934 w1007 w1062 w1092 w1143 w1193 w1282 w1353 w1400 w1455] -> w158
      tunnel: [w198 w225 w254 w313 w397 w459 w542 w619 w689 w722 w758 w791 w819 w833 w859 w897 w935 w1008 w1063 w1093 w1144 w1194 w1283 w1354 w1401 w1456] -> w157
      tunnel: [w197 w224 w253 w312 w396 w458 w545 w622 w688 w721 w757 w790 w806 w839 w858 w898 w936 w1009 w1064 w1094 w1145 w1195 w1284 w1355 w1402 w1457] -> w156
      tunnel: w155 -> [_ _ _ w307 w393 _ w538 _ _ _ _ _ _ _ _ _ _ _ _ _ _ _ _ _ _ _]
      tunnel: w154 -> [_ _ _ w305 w392 _ _ _ _ _ _ _ _ _ _ _ _ _ _ _ _ _ _ _ _ _]
      tunnel: [w196 w220 w246 w282 w369 w448 w535 w608 w683 w715 w751 w776 w804 w832 w857 w879 w925 w990 w1055 w1080 w1135 w1186 w1235 w1310 w1391 w1447] -> w125
      tunnel: w153 -> [w196 w220 w246 w296 w369 w448 w535 w608 w683 w715 w751 w776 w804 w832 w857 w879 w925 w990 w1055 w1080 w1135 w1186 w1235 w1310 w1391 w1447]
      tunnel: w115 -> [_ _ _ w292 w366 w446 w532 w605 _ _ _ _ _ _ _ w877 w923 w987 _ w1077 w1132 w1183 w1232 w1306 _ _]
      tunnel: w151 -> [_ _ _ w289 w365 w444 w531 w604 _ _ _ _ _ _ _ w875 w921 w986 _ w1076 w1131 w1182 w1231 w1307 _ w1415]
      tunnel: w77 -> [_ _ _ w283 _ _ _ _ _ _ _ _ _ _ _ _ _ _ _ _ _ _ _ _ _ w1418]
      tunnel: [w195 w219 w245 w280 w368 w447 w534 w607 w682 w714 w750 w775 w803 w831 w856 w878 w924 w989 w1054 w1079 w1134 w1185 w1234 w1309 w1397 w1427] -> w79
      tunnel: w149 -> [w195 w219 w245 w288 w368 w447 w534 w607 w682 w714 w750 w775 w803 w831 w856 w878 w924 w989 w1054 w1079 w1134 w1185 w1234 w1309 w1397 w1427]
      tunnel: [w194 w218 w244 w278 w364 w443 w530 w603 w681 w713 w749 w774 w802 w830 w855 w874 w920 w985 w1053 w1075 w1130 w1181 w1230 w1305 w1386 w1443] -> w120
      tunnel: w121 -> [w194 w218 w244 w277 w364 w443 w530 w603 w681 w713 w749 w774 w802 w830 w855 w874 w920 w985 w1053 w1075 w1130 w1181 w1230 w1305 w1386 w1443]
      tunnel: [w193 w217 w243 w270 w363 w442 w520 w602 w680 w712 w748 w773 w801 w829 w854 w873 w919 w984 w1052 w1074 w1129 w1180 w1229 w1304 w1385 w1442] -> w103
      tunnel: w106 -> [w193 w217 w243 w270 w363 w442 w520 w602 w680 w712 w748 w773 w801 w829 w854 w873 w919 w984 w1052 w1074 w1129 w1180 w1229 w1304 w1384 w1416]
      tunnel: [w192 w216 w242 w269 w362 w441 w519 w601 w679 w711 w747 w772 w800 w828 w853 w872 w918 w983 w1051 w1073 w1128 w1179 w1228 w1303 w1370 w1429] -> w80
      tunnel: w98 -> [w192 w216 w242 w269 w362 w441 w519 w601 w679 w711 w747 w772 w800 w828 w853 w872 w918 w983 w1051 w1073 w1128 w1179 w1228 w1303 w1370 w1428]
      tunnel: [w191 w215 w241 w268 w361 w440 w518 w600 w678 w710 w746 w771 w799 w827 w852 w871 w917 w982 w1050 w1072 w1127 w1178 w1227 w1302 w1369 w1411] -> w58
      tunnel: w97 -> [w191 w215 w241 w268 w361 w440 w518 w600 w678 w710 w746 w771 w799 w827 w852 w871 w917 w982 w1050 w1072 w1127 w1178 w1227 w1302 w1369 w1409]
      tunnel: [w190 w214 w240 w267 w360 w439 w517 w599 w677 w709 w745 w770 w798 w826 w851 w870 w916 w981 w1049 w1071 w1126 w1177 w1226 w1301 w1368 w1408] -> w96
      tunnel: w95 -> [w190 w214 w240 w267 w360 w439 w517 w599 w677 w709 w745 w770 w798 w826 w851 w870 w916 w981 w1049 w1071 w1126 w1177 w1226 w1301 w1368 w1419]
      tunnel: w77 -> [_ _ _ _ _ _ _ _ _ _ _ _ _ _ _ _ _ _ _ _ _ _ _ _ _ w1407]
      tunnel: w76 -> [w189 w213 w239 w266 w359 w438 w516 w598 w676 w708 w744 w769 w797 w825 w850 w869 w915 w980 w1048 w1070 w1125 w1176 w1225 w1300 w1367 w1406]
      tunnel: [w189 w213 w239 w266 w359 w438 w516 w598 w676 w708 w744 w769 w797 w825 w850 w869 w915 w980 w1048 w1070 w1125 w1176 w1225 w1300 w1367 w1405] -> w51
      tunnel: [w188 w212 w238 w265 w358 w437 w515 w597 w675 w707 w743 w768 w796 w824 w849 w868 w914 w979 w1047 w1069 w1124 w1175 w1224 w1299 w1366 w1404] -> w50
      tunnel: w57 -> [w188 w212 w238 w265 w358 w437 w515 w597 w675 w707 w743 w768 w796 w824 w849 w868 w914 w979 w1047 w1069 w1124 w1175 w1224 w1299 w1366 w1403]
      frame "wait" {
        n29 = Index Array(array=w211, index=0 ("Index")) -> (element=w209:string)
        n30 = Decimal String To Number(string=w209, default (0L)=u32 0) -> (number=w208:u32)  [unwired: 1 in, 1 out]
        n31 = Wait (ms)(milliseconds to wait=w208) -> ()  [unwired: 1 out]
      }
      frame "wait-min" {
        n32 = Index Array(array=w237, index=0 ("Index")) -> (element=w235:string)
        n33 = Decimal String To Number(string=w235, default (0L)=u32 0) -> (number=w223:u32)  [unwired: 1 in, 1 out]
        n34 = Multiply(x=w223, y=u32 60000) -> (x*y=w222:u32)
        n35 = Wait (ms)(milliseconds to wait=w222) -> ()  [unwired: 1 out]
      }
      frame "standby" {
        n36 = Index Array(array=w262, index=0 ("Index")) -> (element=w252:string)
        n37 = case shown="\"on\"" w252 {
          tunnel: [":PAGE:SCON:STAN 0" ":PAGE:SCON:STAN 1"] -> w247
          frame "off", Default {
          }
          frame "on" {
          }
        }
        n38 = VISA Write(VISA resource name=w251, write buffer=w247, error in (no error)=w250) -> (VISA resource name out=w249:refnum<visa-resource-name>, error out=w248:errorcluster)  [unwired: 1 out]
      }
      frame "transfer" {
        # "Don't connect the error lines\nof the two Split blocks!"
        # "Adjusts graph colors."
        # "Time array"
        n39 = Bundle By Name(cluster=w305, "Emergency Stop"=w354) -> (w306:T2)
        n40 = Number To Decimal String(number=w292) -> (decimal integer string=w291:string)  [unwired: 1 in]
        n41 = Delete From Array(array=w344, index=0 ("Index")) -> (deleted portion=w342:string, array with subset deleted=w341:string[])  [unwired: 1 in]
        n42 = Concatenate Strings(w351, "Prefix (transfer)", w291, w289, "Suffix (transfer)") -> (w353:string)
        n43 = VISA Write(VISA resource name=w322, write buffer=":PAGE:CHAN:MODE SWE;" ("write buffer (\"\")"), error in (no error)=w321) -> (VISA resource name out=w319:refnum<visa-resource-name>, error out=w320:errorcluster)  [unwired: 1 out]
        n44 = case shown="\"d\", Default" w342 {
          tunnel: [w356 w357] -> w340
          frame "s" {
            w356 = u16 0 items=["Single", "Double"] ("sweep mode")
          }
          frame "d", Default {
            w357 = u16 1 items=["Single", "Double"] ("sweep mode")
          }
        }
        n45 = String To Path(string=w353) -> (path=w350:path)
        n46 = Fract/Exp String To Number(string=w341) -> (number=w326:dbl[])  [unwired: 3 in, 1 out]
        n47 = Index Array(array=w326, index #1=0 ("Index")) -> (element #1=w339:dbl, element #2=w338:dbl, element #3=w337:dbl)  [unwired: 2 in]
        n48 = Delete From Array(array=w326, length=3 ("Length"), index=0 ("Index")) -> (array with subset deleted=w324:dbl[])  [unwired: 1 out]
        n49 = Build Array (concatenate)(w288, w283) -> (w280:i32[])
        n50 = Bundle By Name(cluster=w331, "Gate Start"=w339, "Gate Stop"=w338, "Gate Step (linear only)"=w337, "Gate Compliance"=w348, "Range mode"=w315, "Range"=w314) -> (w316:T4)
        n51 = call "4155C Split array.vi"("X data in"=w280, "Y1 data in"=w277) -> ("Array of clusters"=w281:cluster{"Y data in":dbl[], "X data in":dbl[]}[])  [unwired: 5 in, 1 out]
        n52 = local write "Id min vs time"(w281) -> ()
        n53 = Index Array(array=w324, index #1=0 ("Index")) -> (element #1=w334:dbl, element #2=w333:dbl, element #3=w332:dbl)  [unwired: 2 in]
        n54 = call <vilib>:"compatOverwrite.vi"("overwrite (F)"=TRUE) -> ("overwrite?"=w304:T7)
        n55 = control-ref of="I vs Vg"() -> (w293:refnum<vi>)
        n56 = Bundle By Name(cluster=w330, "Drain Start"=w334, "Drain Stop"=w333, "Drain Step"=w332, "Drain Compliance"=w349, "Range mode"=w313, "Range"=w312) -> (w317:T5)
        n57 = call "4155C Transfer.vi"("VISA resource name in"=w319, "Gate"=w316, "Drain"=w317, "Timings"=w347, "error in (no error)"=w320, "SMU4"=w307, "sweep mode"=w340, "Panel Controls"=w306) -> ("VG"=w297:dbl[], "Outparams"=w311:T8, "VISA Resource Name out"=w346:refnum<visa-resource-name>, "IS"=w298:dbl[], "ID"=w303:dbl[], "IG"=w299:dbl[], "error out"=w284:errorcluster, "SMU4"=w308:dbl[])  [unwired: 12 in]
        n58 = Unbundle By Name(w311) -> ("V2 Step"=w310:dbl, "V2 Start"=w309:dbl, "Number of points"=w294:i32)
        n59 = call "4155C Split array.vi"("Number of VAR2 steps"=w294, "Y2 data in"=w303, "X data in"=w297, "Y1 data in"=w298, "Y3 data in"=w299, "error in (no error)"=w284) -> ("Array of clusters"=w287:cluster{"Y data in":dbl[], "X data in":dbl[]}[], "error out"=w285:errorcluster)  [unwired: 1 in]
        n60 = local write "I vs Vg"(w287) -> ()
        n61 = Absolute Value(x=w298) -> (abs(x)=w302:dbl[])
        n62 = Array Max & Min(array=w298) -> (max value=w300:dbl)  [unwired: 3 out]
        n63 = Array Max & Min(array=w299) -> (max value=w301:dbl)  [unwired: 3 out]
        n64 = local write "Is"(w300) -> ()
        n65 = Array Max & Min(array=w302) -> (max value=w295:dbl, min value=w279:dbl)  [unwired: 2 out]
        n66 = local write "Ig"(w301) -> ()
        n67 = Build Array (concatenate)(w296, w295) -> (w282:dbl[])
        n68 = call "4155C Split array.vi"("X data in"=w280, "Y1 data in"=w282) -> ("Array of clusters"=w286:cluster{"Y data in":dbl[], "X data in":dbl[]}[])  [unwired: 5 in, 1 out]
        n69 = local write "Id max vs time"(w286) -> ()
        n70 = local write "Id"(w295) -> ()
        n71 = Open/Create/Replace File(file path (use dialog)=w350, error in=w285, operation (0:open)=w304) -> (refnum out=w275:refnum<file>, error out=w273:errorcluster)  [unwired: 3 in, 1 out]
        n72 = call "4155C Make Big 2d array.vi"("1D Var1"=w297, "1d IS"=w298, "1d ID"=w303, "1d IG"=w299, "1d SMU4"=w308, "SMU4"=w307, "VAR2 START"=w309, "Number of VAR2 steps"=w294, "VAR2 STEP"=w310, "VAR1 Name"="Vg", "Decimal places in header"=i8 1, "VAR2 Name"="Vd") -> ("Header array"=w276:string[], "Data array"=w274:dbl[][])  [unwired: 14 in]
        n73 = call "4155C Config Chart Colours.vi"("Numeric"=w294, "XY Graph 2"=w293) -> ()  [unwired: 6 in]
        n74 = call "4155C Write array to file.vi"("Byte Stream File Refnum"=w275, "Header"=w276, "Data Array"=w274, "error in (no error)"=w273) -> ("dup refnum"=w272:refnum<file>, "error out"=w271:errorcluster)  [unwired: 1 in]
        n75 = Build Array (concatenate)(w277, w279) -> (w278:dbl[])
        n76 = Close File(refnum=w272, error in=w271) -> (error out=w345:errorcluster)  [unwired: 1 out]
      }
      frame "pulsedstressV" {
        w375 = 0
        n77 = Number To Decimal String(number=w366) -> (decimal integer string=w423:string)  [unwired: 1 in]
        n78 = Delete From Array(array=w415, index=0 ("Index")) -> (deleted portion=w413:string, array with subset deleted=w412:string[])  [unwired: 1 in]
        n79 = Bundle By Name(cluster=w392, "Emergency Stop"=w426) -> (w394:T2)
        n80 = VISA Write(VISA resource name=w406, write buffer=":PAGE:CHAN:MODE SWE;" ("write buffer (\"\")"), error in (no error)=w405) -> (VISA resource name out=w403:refnum<visa-resource-name>, error out=w404:errorcluster)  [unwired: 1 out]
        n81 = Concatenate Strings(w422, "-pulsedstressV-" ("Substring"), w423, w365, ".txt" ("Substring")) -> (w425:string)
        n82 = case shown="\"d\", Default" w413 {
          tunnel: [w435 w436] -> w411
          frame "s" {
            w435 = u16 0 items=["Single", "Double"] ("sweep mode")
          }
          frame "d", Default {
            w436 = u16 1 items=["Single", "Double"] ("sweep mode")
          }
        }
        n83 = Fract/Exp String To Number(string=w412) -> (number=w407:dbl[])  [unwired: 3 in, 1 out]
        n84 = String To Path(string=w425) -> (path=w421:path)
        n85 = Index Array(array=w407, index #1=0 ("Index")) -> (element #1=w384:dbl, element #2=w383:dbl, element #3=w380:dbl, element #4=w379:dbl, element #5=w378:dbl, element #6=w382:dbl)  [unwired: 5 in]
        n86 = Bundle By Name(cluster=w381, "Pulse period"=w379, "Base voltage"=w380, "Pulse width"=w378) -> (w377:T6)
        n87 = Unbundle By Name(w377) -> ("Pulse period"=w385:dbl)
        n88 = Bundle By Name(cluster=w409, "Gate Start"=w383, "Gate Stop"=w384, "Gate Step (linear only)"=0, "Gate Compliance"=w419, "Range mode"=w399, "Range"=w398) -> (w400:T4)
        n89 = call <vilib>:"compatOverwrite.vi"("overwrite (F)"=TRUE) -> ("overwrite?"=w370:T7)
        n90 = Bundle By Name(cluster=w408, "Drain Start"=w382, "Drain Stop"=w375, "Drain Step"=w375, "Drain Compliance"=w420, "Range mode"=w397, "Range"=w396) -> (w401:T5)
        n91 = call "4155C PulsedStressV.vi"("VISA resource name in"=w403, "sweep mode"=w411, "Panel Controls"=w394, "Gate"=w400, "Drain"=w401, "Timings"=w377, "error in (no error)"=w404, "SMU4"=w393) -> ("VISA Resource Name out"=w417:refnum<visa-resource-name>, "ID"=w373:dbl[], "IG"=w371:dbl[], "Outparams"=w395:T8, "error out"=w418:errorcluster)  [unwired: 3 in]
        n92 = Unbundle By Name(w395) -> ("Number of points"=w372:i32)  [unwired: 2 out]
        n93 = for {
          N: w372 -> [_]
          tunnel: [w432] -> w374 mode=indexing
          tunnel: w385 -> [w434]
          i -> [w433]
          n94 = Multiply(x=w434, y=w433) -> (x*y=w432:dbl)
        }
        n95 = Insert Into Array(array=dbl[][] [] ("Input Array"), new element=w374) -> (w386:dbl[][])  [unwired: 2 in]
        n96 = Insert Into Array(array=w386, new element=w373) -> (w391:dbl[][])  [unwired: 2 in]
        n97 = Insert Into Array(array=w391, new element=w371) -> (w390:dbl[][])  [unwired: 2 in]
        n98 = Transpose 2D Array(2D array=w390) -> (transposed array=w389:dbl[][])
        n99 = Open/Create/Replace File(file path (use dialog)=w421, error in=w418, operation (0:open)=w370) -> (refnum out=w429:refnum<file>, error out=w430:errorcluster)  [unwired: 3 in, 1 out]
        n100 = call "4155C Write array to file.vi"("Byte Stream File Refnum"=w429, "Header"=string[] ["Time /s", "Id /A", "Ig /A"], "Data Array"=w389, "error in (no error)"=w430) -> ("dup refnum"=w427:refnum<file>, "error out"=w428:errorcluster)  [unwired: 1 in]
        n101 = Close File(refnum=w427, error in=w428) -> (error out=w416:errorcluster)  [unwired: 1 out]
      }
      frame "transfer-fpp" {
        n102 = Number To Decimal String(number=w446) -> (decimal integer string=w500:string)  [unwired: 1 in]
        n103 = Bundle By Name(cluster=w476, "Emergency Stop"=w504) -> (w512:T1)
        n104 = Delete From Array(array=w491, index=0 ("Index")) -> (deleted portion=w489:string, array with subset deleted=w488:string[])  [unwired: 1 in]
        n105 = Concatenate Strings(w499, "-transferfpp-" ("Substring"), w500, w444, ".txt" ("Substring")) -> (w502:string)
        n106 = VISA Write(VISA resource name=w468, write buffer=":PAGE:CHAN:MODE SWE;" ("write buffer (\"\")"), error in (no error)=w467) -> (VISA resource name out=w465:refnum<visa-resource-name>, error out=w466:errorcluster)  [unwired: 1 out]
        n107 = case shown="\"d\", Default" w489 {
          tunnel: [w513 w514] -> w487
          frame "s" {
            w513 = u16 0 items=["Single", "Double"] ("sweep mode")
          }
          frame "d", Default {
            w514 = u16 1 items=["Single", "Double"] ("sweep mode")
          }
        }
        n108 = Fract/Exp String To Number(string=w488) -> (number=w472:dbl[])  [unwired: 3 in, 1 out]
        n109 = String To Path(string=w502) -> (path=w498:path)
        n110 = Index Array(array=w472, index #1=0 ("Index")) -> (element #1=w486:dbl, element #2=w485:dbl, element #3=w484:dbl)  [unwired: 2 in]
        n111 = Delete From Array(array=w472, length=3 ("Length"), index=0 ("Index")) -> (array with subset deleted=w470:dbl[])  [unwired: 1 out]
        n112 = Bundle By Name(cluster=w478, "Gate Start"=w486, "Gate Stop"=w485, "Gate Step (linear only)"=w484, "Gate Compliance"=w496, "Range mode"=w461, "Range"=w460) -> (w462:T4)
        n113 = Index Array(array=w470, index #1=0 ("Index")) -> (element #1=w481:dbl, element #2=w480:dbl, element #3=w479:dbl)  [unwired: 2 in]
        n114 = call <vilib>:"compatOverwrite.vi"("overwrite (F)"=TRUE) -> ("overwrite?"=w449:T7)
        n115 = Bundle By Name(cluster=w477, "Drain Start"=w481, "Drain Stop"=w480, "Drain Step"=w479, "Drain Compliance"=w497, "Range mode"=w459, "Range"=w458) -> (w463:T5)
        n116 = call "4155C Transfer-FPP.vi"("VISA resource name in"=w465, "Gate"=w462, "Drain"=w463, "Timings"=w495, "error in (no error)"=w466, "sweep mode"=w487, "Panel Controls"=w512) -> ("VG"=w503:dbl[], "Outparams"=w457:T8, "VISA Resource Name out"=w493:refnum<visa-resource-name>, "Vprobe2"=w453:dbl[], "ID"=w452:dbl[], "IG"=w451:dbl[], "Vprobe1"=w450:dbl[], "error out"=w494:errorcluster)  [unwired: 13 in]
        n117 = Unbundle By Name(w457) -> ("V2 Step"=w456:dbl, "V2 Start"=w455:dbl, "Number of points"=w454:i32)
        n118 = Open/Create/Replace File(file path (use dialog)=w498, error in=w494, operation (0:open)=w449) -> (refnum out=w509:refnum<file>, error out=w510:errorcluster)  [unwired: 3 in, 1 out]
        n119 = call "4155C Make Big 2d array FPP.vi"("1D Var1"=w503, "1d ID"=w452, "1d Vp2"=w453, "1d IG"=w451, "1d Vp1"=w450, "VAR2 START"=w455, "Number of VAR2 steps"=w454, "VAR2 STEP"=w456, "VAR1 Name"="Vg", "Decimal places in header"=i8 1, "VAR2 Name"="Vd") -> ("Header array"=w505:string[], "Data array"=w506:dbl[][])  [unwired: 15 in]
        n120 = call "4155C Write array to file.vi"("Byte Stream File Refnum"=w509, "Header"=w505, "Data Array"=w506, "error in (no error)"=w510) -> ("dup refnum"=w507:refnum<file>, "error out"=w508:errorcluster)  [unwired: 1 in]
        n121 = Close File(refnum=w507, error in=w508) -> (error out=w492:errorcluster)  [unwired: 1 out]
      }
      frame "output" {
        n122 = Number To Decimal String(number=w532) -> (decimal integer string=w581:string)  [unwired: 1 in]
        n123 = Bundle By Name(cluster=w558, "Emergency Stop"=w584) -> (w594:T1)
        n124 = Delete From Array(array=w573, index=0 ("Index")) -> (deleted portion=w571:string, array with subset deleted=w570:string[])  [unwired: 1 in]
        n125 = Concatenate Strings(w580, "Prefix (output)", w581, w531, "Suffix (output)") -> (w583:string)
        n126 = VISA Write(VISA resource name=w549, write buffer=":PAGE:CHAN:MODE SWE;" ("write buffer (\"\")"), error in (no error)=w546) -> (VISA resource name out=w548:refnum<visa-resource-name>, error out=w547:errorcluster)  [unwired: 1 out]
        n127 = case shown="\"d\", Default" w571 {
          tunnel: [w595 w596] -> w569
          frame "s" {
            w595 = u16 0 items=["Single", "Double"] ("sweep mode")
          }
          frame "d", Default {
            w596 = u16 1 items=["Single", "Double"] ("sweep mode")
          }
        }
        n128 = Fract/Exp String To Number(string=w570) -> (number=w552:dbl[])  [unwired: 3 in, 1 out]
        n129 = String To Path(string=w583) -> (path=w579:path)
        n130 = Index Array(array=w552, index #1=0 ("Index")) -> (element #1=w568:dbl, element #2=w567:dbl, element #3=w566:dbl)  [unwired: 2 in]
        n131 = Delete From Array(array=w552, length=3 ("Length"), index=0 ("Index")) -> (array with subset deleted=w551:dbl[])  [unwired: 1 out]
        n132 = control-ref of="I vs Vd"() -> (w522:refnum<vi>)
        n133 = Bundle By Name(cluster=w560, "Gate Start"=w568, "Gate Stop"=w567, "Gate Step (linear only)"=w566, "Gate Compliance"=w577, "Range mode"=w544, "Range"=w543) -> (w593:T4)
        n134 = Index Array(array=w551, index #1=0 ("Index")) -> (element #1=w563:dbl, element #2=w562:dbl, element #3=w561:dbl)  [unwired: 2 in]
        n135 = call <vilib>:"compatOverwrite.vi"("overwrite (F)"=TRUE) -> ("overwrite?"=w536:T7)
        n136 = Bundle By Name(cluster=w559, "Drain Start"=w563, "Drain Stop"=w562, "Drain Step"=w561, "Drain Compliance"=w578, "Range mode"=w542, "Range"=w545) -> (w592:T5)
        n137 = call "4155C Output.vi"("VISA resource name in"=w548, "Gate"=w593, "Drain"=w592, "Timings"=w576, "error in (no error)"=w547, "SMU4"=w538, "sweep mode"=w569, "Panel controls"=w594) -> ("VD"=w529:dbl[], "Outparams"=w540:T8, "VISA Resource Name out"=w575:refnum<visa-resource-name>, "IS"=w528:dbl[], "ID"=w527:dbl[], "IG"=w526:dbl[], "error out"=w524:errorcluster, "SMU4"=w537:dbl[])  [unwired: 12 in]
        n138 = Unbundle By Name(w540) -> ("V2 Step"=w541:dbl, "V2 Start"=w539:dbl, "Number of points"=w521:i32)
        n139 = call "4155C Split array.vi"("Number of VAR2 steps"=w521, "Y2 data in"=w527, "X data in"=w529, "Y1 data in"=w528, "Y3 data in"=w526, "error in (no error)"=w524) -> ("Array of clusters"=w525:cluster{"Y data in":dbl[], "X data in":dbl[]}[], "error out"=w523:errorcluster)  [unwired: 1 in]
        n140 = local write "I vs Vd"(w525) -> ()
        n141 = call "4155C Config Chart Colours.vi"("Numeric"=w521, "XY Graph 2"=w522) -> ()  [unwired: 6 in]
        n142 = Open/Create/Replace File(file path (use dialog)=w579, error in=w523, operation (0:open)=w536) -> (refnum out=w589:refnum<file>, error out=w590:errorcluster)  [unwired: 3 in, 1 out]
        n143 = call "4155C Make Big 2d array.vi"("1D Var1"=w529, "1d IS"=w528, "1d ID"=w527, "1d IG"=w526, "1d SMU4"=w537, "SMU4"=w538, "VAR2 START"=w539, "Number of VAR2 steps"=w521, "VAR2 STEP"=w541, "VAR1 Name"="Vd", "Decimal places in header"=i8 1, "VAR2 Name"="Vg") -> ("Header array"=w585:string[], "Data array"=w586:dbl[][])  [unwired: 14 in]
        n144 = call "4155C Write array to file.vi"("Byte Stream File Refnum"=w589, "Header"=w585, "Data Array"=w586, "error in (no error)"=w590) -> ("dup refnum"=w587:refnum<file>, "error out"=w588:errorcluster)  [unwired: 1 in]
        n145 = Close File(refnum=w587, error in=w588) -> (error out=w574:errorcluster)  [unwired: 1 out]
      }
      frame "output-fpp" {
        n146 = Number To Decimal String(number=w605) -> (decimal integer string=w659:string)  [unwired: 1 in]
        n147 = Bundle By Name(cluster=w635, "Emergency Stop"=w662) -> (w672:T1)
        n148 = Delete From Array(array=w650, index=0 ("Index")) -> (deleted portion=w648:string, array with subset deleted=w647:string[])  [unwired: 1 in]
        n149 = VISA Write(VISA resource name=w626, write buffer=":PAGE:CHAN:MODE SWE;" ("write buffer (\"\")"), error in (no error)=w623) -> (VISA resource name out=w625:refnum<visa-resource-name>, error out=w624:errorcluster)  [unwired: 1 out]
        n150 = Concatenate Strings(w658, "-outputfpp-" ("Substring"), w659, w604, ".txt" ("Substring")) -> (w661:string)
        n151 = case shown="\"d\", Default" w648 {
          tunnel: [w673 w674] -> w646
          frame "s" {
            w673 = u16 0 items=["Single", "Double"] ("sweep mode")
          }
          frame "d", Default {
            w674 = u16 1 items=["Single", "Double"] ("sweep mode")
          }
        }
        n152 = Fract/Exp String To Number(string=w647) -> (number=w629:dbl[])  [unwired: 3 in, 1 out]
        n153 = String To Path(string=w661) -> (path=w657:path)
        n154 = Index Array(array=w629, index #1=0 ("Index")) -> (element #1=w645:dbl, element #2=w644:dbl, element #3=w643:dbl)  [unwired: 2 in]
        n155 = Delete From Array(array=w629, length=3 ("Length"), index=0 ("Index")) -> (array with subset deleted=w628:dbl[])  [unwired: 1 out]
        n156 = Bundle By Name(cluster=w637, "Gate Start"=w645, "Gate Stop"=w644, "Gate Step (linear only)"=w643, "Gate Compliance"=w655, "Range mode"=w621, "Range"=w620) -> (w671:T4)
        n157 = Index Array(array=w628, index #1=0 ("Index")) -> (element #1=w640:dbl, element #2=w639:dbl, element #3=w638:dbl)  [unwired: 2 in]
        n158 = call <vilib>:"compatOverwrite.vi"("overwrite (F)"=TRUE) -> ("overwrite?"=w609:T7)
        n159 = Bundle By Name(cluster=w636, "Drain Start"=w640, "Drain Stop"=w639, "Drain Step"=w638, "Drain Compliance"=w656, "Range mode"=w619, "Range"=w622) -> (w670:T5)
        n160 = call "4155C Output-FPP.vi"("VISA resource name in"=w625, "Gate"=w671, "Drain"=w670, "Timings"=w654, "error in (no error)"=w624, "sweep mode"=w646, "Panel controls"=w672) -> ("VD"=w614:dbl[], "Outparams"=w617:T8, "VISA Resource Name out"=w652:refnum<visa-resource-name>, "Vprobe2"=w613:dbl[], "ID"=w612:dbl[], "IG"=w611:dbl[], "Vprobe1"=w610:dbl[], "error out"=w653:errorcluster)  [unwired: 13 in]
        n161 = Unbundle By Name(w617) -> ("V2 Step"=w618:dbl, "V2 Start"=w616:dbl, "Number of points"=w615:i32)
        n162 = Open/Create/Replace File(file path (use dialog)=w657, error in=w653, operation (0:open)=w609) -> (refnum out=w667:refnum<file>, error out=w668:errorcluster)  [unwired: 3 in, 1 out]
        n163 = call "4155C Make Big 2d array FPP.vi"("1D Var1"=w614, "1d ID"=w612, "1d Vp2"=w613, "1d IG"=w611, "1d Vp1"=w610, "VAR2 START"=w616, "Number of VAR2 steps"=w615, "VAR2 STEP"=w618, "VAR1 Name"="Vd", "Decimal places in header"=i8 1, "VAR2 Name"="Vg") -> ("Header array"=w663:string[], "Data array"=w664:dbl[][])  [unwired: 15 in]
        n164 = call "4155C Write array to file.vi"("Byte Stream File Refnum"=w667, "Header"=w663, "Data Array"=w664, "error in (no error)"=w668) -> ("dup refnum"=w665:refnum<file>, "error out"=w666:errorcluster)  [unwired: 1 in]
        n165 = Close File(refnum=w665, error in=w666) -> (error out=w651:errorcluster)  [unwired: 1 out]
      }
      frame "itime" {
        n166 = Delete From Array(array=w695, index=0 ("Index")) -> (deleted portion=w696:string)  [unwired: 1 in, 1 out]
        n167 = case shown="\"l\"" w696 {
          tunnel: w694 -> [w700 w702 w705]
          tunnel: [w699 w701 w704] -> w687
          frame "s" {
            w698 = u32 0 items=["short  ", "medium  ", "long  "] ("integration time 2")
            n168 = Bundle By Name(cluster=w700, "integration time"=w698) -> (w699:T6)
          }
          frame "m", Default {
            w703 = u32 1 items=["short  ", "medium  ", "long  "] ("integration time 2")
            n169 = Bundle By Name(cluster=w702, "integration time"=w703) -> (w701:T6)
          }
          frame "l" {
            w706 = u32 2 items=["short  ", "medium  ", "long  "] ("integration time 2")
            n170 = Bundle By Name(cluster=w705, "integration time"=w706) -> (w704:T6)
          }
        }
      }
      frame "pulsed" {
        n171 = Delete From Array(array=w728, index=0 ("Index")) -> (deleted portion=w729:string, array with subset deleted=w716:string[])  [unwired: 1 in]
        n172 = case shown="\"on\", Default" w729 {
          tunnel: w727 -> [w739 w742]
          tunnel: [w738 w741] -> w720
          tunnel: w716 -> [w736 _]
          frame "on", Default {
            w737 = u16 1 items=["Continuous", "Pulsed"] ("sweep method")
            n173 = Fract/Exp String To Number(string=w736) -> (number=w734:dbl[])  [unwired: 3 in, 1 out]
            n174 = Index Array(array=w734, index #1=0 ("Index")) -> (element #1=w733:dbl, element #2=w732:dbl, element #3=w731:dbl)  [unwired: 2 in]
            n175 = Bundle By Name(cluster=w739, "sweep method"=w737, "Pulse period"=w733, "Base voltage"=w732, "Pulse width"=w731) -> (w738:T6)
          }
          frame "off" {
            w740 = u16 0 items=["Continuous", "Pulsed"] ("sweep method")
            n176 = Bundle By Name(cluster=w742, "sweep method"=w740) -> (w741:T6)
          }
        }
      }
      frame "gaterangemode" {
        n177 = Delete From Array(array=w762, index=0 ("Index")) -> (deleted portion=w763:string)  [unwired: 1 in, 1 out]
        n178 = case shown="\"f\"" w763 {
          tunnel: [w765 w766 w767] -> w752
          frame "a", Default {
            w765 = u16 0 items=["Auto", "Limited", "Fixed"] ("Gate Range\nmode 2")
          }
          frame "f" {
            w766 = u16 2 items=["Auto", "Limited", "Fixed"] ("Gate Range\nmode 2")
          }
          frame "l" {
            w767 = u16 1 items=["Auto", "Limited", "Fixed"] ("Gate Range\nmode 2")
          }
        }
      }
      frame "gaterange" {
        (unwired) u8 11 items=["10fA  ", "100fA  ", "1nA  ", "10nA", "100nA", "1uA", "10uA", "100uA", "1mA", "10mA", "100mA", "1A"] ("Gate Range 2")
        n179 = Delete From Array(array=w794, index=0 ("Index")) -> (deleted portion=w784:string)  [unwired: 1 in, 1 out]
        n180 = Scan Value(string=w784, format string="") -> (value=w782:dbl)  [unwired: 1 in, 1 out]
        n181 = Logarithm Base 10(1:w782) -> (0:w781:dbl)
        n182 = Round To Nearest(number=w781) -> (nearest integer value=w780:dbl)
        n183 = Add(x=w780, y=11.0) -> (x+y=w778:dbl)
        n184 = To Unsigned Byte Integer(number=w778) -> (unsigned 8bit integer=w777:u8)
      }
      frame "drainrange" {
        (unwired) u8 11 items=["10fA  ", "100fA  ", "1nA  ", "10nA", "100nA", "1uA", "10uA", "100uA", "1mA", "10mA", "100mA", "1A"] ("Gate Range 2")
        n185 = Delete From Array(array=w822, index=0 ("Index")) -> (deleted portion=w813:string)  [unwired: 1 in, 1 out]
        n186 = Scan Value(string=w813, format string="") -> (value=w811:dbl)  [unwired: 1 in, 1 out]
        n187 = Logarithm Base 10(1:w811) -> (0:w810:dbl)
        n188 = Round To Nearest(number=w810) -> (nearest integer value=w809:dbl)
        n189 = Add(x=w809, y=11.0) -> (x+y=w807:dbl)
        n190 = To Unsigned Byte Integer(number=w807) -> (unsigned 8bit integer=w806:u8)
      }
      frame "drainrangemode" {
        n191 = Delete From Array(array=w843, index=0 ("Index")) -> (deleted portion=w844:string)  [unwired: 1 in, 1 out]
        n192 = case shown="\"f\"" w844 {
          tunnel: [w846 w847 w848] -> w833
          frame "a", Default {
            w846 = u16 0 items=["Auto", "Limited", "Fixed"] ("Gate Range\nmode 2")
          }
          frame "f" {
            w847 = u16 2 items=["Auto", "Limited", "Fixed"] ("Gate Range\nmode 2")
          }
          frame "l" {
            w848 = u16 1 items=["Auto", "Limited", "Fixed"] ("Gate Range\nmode 2")
          }
        }
      }
      frame "Error", Default {
      }
      frame "logfile" {
        n193 = Number To Decimal String(number=w877) -> (decimal integer string=w912:string)  [unwired: 1 in]
        n194 = Concatenate Strings(w911, "logfile" ("Substring"), w912, w875, ".txt" ("Substring")) -> (w909:string)
        n195 = String To Path(string=w909) -> (path=w882:path)
        n196 = Unbundle(w908) -> ("integration time"=w907:u32, "Short/Long integration time"=w906:dbl, "hold time (sec)"=w905:dbl, "delay time (sec)"=w904:dbl, "Step Time (0 disables)"=w903:dbl, "sweep method"=w902:u16, "Pulse period"=w901:dbl, "Base voltage"=w900:dbl, "Pulse width"=w899:dbl)
        n197 = Build Array(w907, w906, w905, w904, w903, w902, w901, w900, w899, w893, w894, w895, w896, w897, w898) -> (w886:dbl[])
        n198 = Insert Into Array(array=dbl[][] [] ("Input Array"), new element=w886) -> (w885:dbl[][])  [unwired: 2 in]
        n199 = call <vilib>:"compatOverwrite.vi"("overwrite (F)"=TRUE) -> ("overwrite?"=w880:T7)
        n200 = Open/Create/Replace File(file path (use dialog)=w882, error in=w884, operation (0:open)=w880) -> (refnum out=w890:refnum<file>, error out=w889:errorcluster)  [unwired: 3 in, 1 out]
        n201 = call "4155C Write array to file.vi"("Byte Stream File Refnum"=w890, "Header"=string[] ["Int Time", "Short/Long Itime", "Hold time", "Delay time", "Step time", "Sweep method", "Pulse period", "Base Voltage", "Pulse width", "Drain compliance", "Gate compliance", "Gate range mode", "Gate range", "S/D range mode", "S/D range"], "Data Array"=w885, "error in (no error)"=w889) -> ("dup refnum"=w892:refnum<file>, "error out"=w891:errorcluster)  [unwired: 1 in]
        n202 = Close File(refnum=w892, error in=w891) -> (error out=w883:errorcluster)  [unwired: 1 out]
      }
      frame "sample" {
        n203 = Number To Decimal String(number=w923) -> (decimal integer string=w971:string)  [unwired: 1 in]
        n204 = Fract/Exp String To Number(string=w968) -> (number=w929:dbl[])  [unwired: 3 in, 1 out]
        n205 = Concatenate Strings(w946, "-sample-" ("Substring"), w971, w921, ".txt" ("Substring")) -> (w969:string)
        n206 = String To Path(string=w969) -> (path=w950:path)
        n207 = Index Array(array=w929, index=0 ("Index")) -> (element=w966:dbl)
        n208 = Index Array(array=w929, index=2 ("Index")) -> (element=w962:dbl)
        n209 = Index Array(array=w929, index=3 ("Index")) -> (element=w931:dbl)
        n210 = Index Array(array=w929, index=4 ("Index")) -> (element=w928:dbl)
        n211 = call "4155C Config Sampling Measurements.vi"("Sampling interval"=w928, "Sample time"=w931, "Display on/off"=TRUE, "Timings"=w937, "Num Points"=w962, "error in (no error)"=w973, "Drain Compliance"=w972, "Gate Compliance"=w947, "VISA session"=w974) -> ("error out"=w975:errorcluster, "dup VISA resource name"=w976:refnum<visa-resource-name>)  [unwired: 1 in]
        n212 = Index Array(array=w929, index=1 ("Index")) -> (element=w963:dbl)
        n213 = call "4155C Take Sample.vi"("Emergency Stop"=w943, "error in (no error)"=w975, "Vd"=w963, "Vg"=w966, "VISA resource name in"=w976) -> ("error out"=w941:errorcluster, "Id"=w978:dbl[], "Ig"=w952:dbl[], "VISA Resource Name out"=w939:refnum<visa-resource-name>, "Is"=w977:dbl[], "Time"=w956:dbl[])  [unwired: 1 in]
        n214 = Insert Into Array(array=dbl[][] [] ("Input Array"), new element=w956) -> (w955:dbl[][])  [unwired: 2 in]
        n215 = Insert Into Array(array=w955, new element=w952) -> (w954:dbl[][])  [unwired: 2 in]
        n216 = Insert Into Array(array=w954, new element=w978) -> (w953:dbl[][])  [unwired: 2 in]
        n217 = VISA Write(VISA resource name=w939, write buffer=":DISP ON" ("write buffer (\"\")"), error in (no error)=w941) -> (VISA resource name out=w938:refnum<visa-resource-name>, error out=w940:errorcluster)  [unwired: 1 out]
        n218 = Insert Into Array(array=w953, new element=w977) -> (w945:dbl[][])  [unwired: 2 in]
        n219 = Transpose 2D Array(2D array=w945) -> (transposed array=w944:dbl[][])
        n220 = call <vilib>:"compatOverwrite.vi"("overwrite (F)"=TRUE) -> ("overwrite?"=w926:T7)
        n221 = Open/Create/Replace File(file path (use dialog)=w950, error in=w940, operation (0:open)=w926) -> (refnum out=w959:refnum<file>, error out=w958:errorcluster)  [unwired: 3 in, 1 out]
        n222 = call "4155C Write array to file.vi"("Byte Stream File Refnum"=w959, "Header"=string[] ["Time /s", "Ig /A", "Id /A", "Is /A"], "Data Array"=w944, "error in (no error)"=w958) -> ("dup refnum"=w961:refnum<file>, "error out"=w960:errorcluster)  [unwired: 1 in]
        n223 = Close File(refnum=w961, error in=w960) -> (error out=w948:errorcluster)  [unwired: 1 out]
      }
      frame "samplei" {
        n224 = Number To Decimal String(number=w987) -> (decimal integer string=w1039:string)  [unwired: 1 in]
        n225 = Fract/Exp String To Number(string=w1036) -> (number=w1003:dbl[])  [unwired: 3 in, 1 out]
        n226 = Concatenate Strings(w1018, "-samplei-" ("Substring"), w1039, w986, ".txt" ("Substring")) -> (w1037:string)
        n227 = String To Path(string=w1037) -> (path=w1021:path)
        n228 = Index Array(array=w1003, index=4 ("Index")) -> (element=w997:dbl)
        n229 = Index Array(array=w1003, index=3 ("Index")) -> (element=w998:dbl)
        n230 = Index Array(array=w1003, index=1 ("Index")) -> (element=w1000:dbl)
        n231 = Index Array(array=w1003, index=0 ("Index")) -> (element=w1001:dbl)
        n232 = Index Array(array=w1003, index=2 ("Index")) -> (element=w999:dbl)
        n233 = call "4155C Config SamplingI Measurements.vi"("Sample time"=w999, "Display on/off"=TRUE, "Timings"=w1010, "Num Points"=w1000, "error in (no error)"=w1041, "Sampling interval"=w998, "VISA session"=w1042) -> ("error out"=w1043:errorcluster, "dup VISA resource name"=w1044:refnum<visa-resource-name>)  [unwired: 3 in]
        n234 = call "4155C Take SampleI.vi"("Emergency Stop"=w1015, "error in (no error)"=w1043, "Idg 2"=w1001, "Vdg compliance 2"=w997, "VISA resource name in"=w1044) -> ("error out"=w1013:errorcluster, "Idg"=w1046:dbl[], "Vdg"=w1023:dbl[], "VISA Resource Name out"=w1011:refnum<visa-resource-name>, "Is"=w1045:dbl[], "Time"=w1027:dbl[])  [unwired: 1 in]
        n235 = Insert Into Array(array=dbl[][] [] ("Input Array"), new element=w1027) -> (w1026:dbl[][])  [unwired: 2 in]
        n236 = Insert Into Array(array=w1026, new element=w1023) -> (w1025:dbl[][])  [unwired: 2 in]
        n237 = Insert Into Array(array=w1025, new element=w1046) -> (w1024:dbl[][])  [unwired: 2 in]
        n238 = VISA Write(VISA resource name=w1011, write buffer=":DISP ON" ("write buffer (\"\")"), error in (no error)=w1013) -> (VISA resource name out=w996:refnum<visa-resource-name>, error out=w1012:errorcluster)  [unwired: 1 out]
        n239 = Insert Into Array(array=w1024, new element=w1045) -> (w1017:dbl[][])  [unwired: 2 in]
        n240 = Transpose 2D Array(2D array=w1017) -> (transposed array=w1016:dbl[][])
        n241 = call <vilib>:"compatOverwrite.vi"("overwrite (F)"=TRUE) -> ("overwrite?"=w991:T7)
        n242 = Open/Create/Replace File(file path (use dialog)=w1021, error in=w1012, operation (0:open)=w991) -> (refnum out=w1030:refnum<file>, error out=w1029:errorcluster)  [unwired: 3 in, 1 out]
        n243 = call "4155C Write array to file.vi"("Byte Stream File Refnum"=w1030, "Header"=string[] ["Time /s", "Vdg /V", "Idg /A", "Is /A"], "Data Array"=w1016, "error in (no error)"=w1029) -> ("dup refnum"=w1032:refnum<file>, "error out"=w1031:errorcluster)  [unwired: 1 in]
        n244 = Close File(refnum=w1032, error in=w1031) -> (error out=w994:errorcluster)  [unwired: 1 out]
        n245 = VISA Write(VISA resource name=w996, write buffer=";:PAGE:SCON:STAN OFF;:PAGE:CHAN:VSU2:DIS;" ("write buffer (\"\")"), error in (no error)=w994) -> (VISA resource name out=w992:refnum<visa-resource-name>, error out=w993:errorcluster)  [unwired: 1 out]
      }
      frame "#" {
        n246 = VISA Write(VISA resource name=w1060, write buffer=":DISP ON" ("write buffer (\"\")"), error in (no error)=w1059) -> (VISA resource name out=w1058:refnum<visa-resource-name>, error out=w1057:errorcluster)  [unwired: 1 out]
      }
      frame "stressV" {
        n247 = Number To Decimal String(number=w1077) -> (decimal integer string=w1118:string)  [unwired: 1 in]
        n248 = Fract/Exp String To Number(string=w1115) -> (number=w1088:dbl[])  [unwired: 3 in, 1 out]
        n249 = Concatenate Strings(w1102, "-stressV-" ("Substring"), w1118, w1076, ".txt" ("Substring")) -> (w1116:string)
        n250 = String To Path(string=w1116) -> (path=w1106:path)
        n251 = Index Array(array=w1088, index=3 ("Index")) -> (element=w1085:dbl)
        n252 = Index Array(array=w1088, index=1 ("Index")) -> (element=w1083:dbl)
        n253 = Index Array(array=w1088, index=0 ("Index")) -> (element=w1082:dbl)
        n254 = Index Array(array=w1088, index=4 ("Index")) -> (element=w1087:dbl)
        n255 = Index Array(array=w1088, index=2 ("Index")) -> (element=w1084:dbl)
        n256 = call "4155C Config V Stress.vi"("VISA session"=w1121, "ID compliance"=w1085, "VD"=w1083, "VG"=w1082, "IG compliance"=w1084, "error in (no error)"=w1120, "Display on/off"=TRUE) -> ("dup VISA resource name"=w1123:refnum<visa-resource-name>, "error out"=w1122:errorcluster)
        n257 = call "4155C Apply Stress.vi"("error in (no error)"=w1122, "Duration"=w1087, "Emergency Stop"=w1101, "VISA resource name in"=w1123) -> ("error out"=w1099:errorcluster, "VISA Resource Name out"=w1097:refnum<visa-resource-name>)
        n258 = VISA Write(VISA resource name=w1097, write buffer=":DISP ON" ("write buffer (\"\")"), error in (no error)=w1099) -> (VISA resource name out=w1096:refnum<visa-resource-name>, error out=w1098:errorcluster)  [unwired: 1 out]
        n259 = call <vilib>:"compatOverwrite.vi"("overwrite (F)"=TRUE) -> ("overwrite?"=w1081:T7)
        n260 = Open/Create/Replace File(file path (use dialog)=w1106, error in=w1098, operation (0:open)=w1081) -> (refnum out=w1109:refnum<file>, error out=w1108:errorcluster)  [unwired: 3 in, 1 out]
        n261 = call "4155C Write array to file.vi"("Byte Stream File Refnum"=w1109, "Header"=string[] ["V stress completed successfully", ""], "error in (no error)"=w1108) -> ("dup refnum"=w1111:refnum<file>, "error out"=w1110:errorcluster)  [unwired: 2 in]
        n262 = Close File(refnum=w1111, error in=w1110) -> (error out=w1104:errorcluster)  [unwired: 1 out]
      }
      frame "stressI" {
        n263 = Number To Decimal String(number=w1132) -> (decimal integer string=w1169:string)  [unwired: 1 in]
        n264 = Fract/Exp String To Number(string=w1166) -> (number=w1141:dbl[])  [unwired: 3 in, 1 out]
        n265 = Concatenate Strings(w1153, "-stressI-" ("Substring"), w1169, w1131, ".txt" ("Substring")) -> (w1167:string)
        n266 = String To Path(string=w1167) -> (path=w1157:path)
        n267 = Index Array(array=w1141, index=1 ("Index")) -> (element=w1137:dbl)
        n268 = Index Array(array=w1141, index=0 ("Index")) -> (element=w1138:dbl)
        n269 = call "4155C Config I Stress.vi"("VISA session"=w1172, "IDG"=w1138, "VDG compliance"=w1137, "error in (no error)"=w1171, "Display on/off"=TRUE) -> ("dup VISA resource name"=w1174:refnum<visa-resource-name>, "error out"=w1173:errorcluster)
        n270 = Index Array(array=w1141, index=2 ("Index")) -> (element=w1139:dbl)
        n271 = call "4155C Apply Stress.vi"("error in (no error)"=w1173, "Duration"=w1139, "Emergency Stop"=w1152, "VISA resource name in"=w1174) -> ("error out"=w1150:errorcluster, "VISA Resource Name out"=w1148:refnum<visa-resource-name>)
        n272 = VISA Write(VISA resource name=w1148, write buffer=":DISP ON" ("write buffer (\"\")"), error in (no error)=w1150) -> (VISA resource name out=w1147:refnum<visa-resource-name>, error out=w1149:errorcluster)  [unwired: 1 out]
        n273 = call <vilib>:"compatOverwrite.vi"("overwrite (F)"=TRUE) -> ("overwrite?"=w1136:T7)
        n274 = Open/Create/Replace File(file path (use dialog)=w1157, error in=w1149, operation (0:open)=w1136) -> (refnum out=w1160:refnum<file>, error out=w1159:errorcluster)  [unwired: 3 in, 1 out]
        n275 = call "4155C Write array to file.vi"("Byte Stream File Refnum"=w1160, "Header"=string[] ["I stress completed successfully", ""], "error in (no error)"=w1159) -> ("dup refnum"=w1162:refnum<file>, "error out"=w1161:errorcluster)  [unwired: 2 in]
        n276 = Close File(refnum=w1162, error in=w1161) -> (error out=w1155:errorcluster)  [unwired: 1 out]
      }
      frame "vsu2pulse" {
        n277 = Number To Decimal String(number=w1183) -> (decimal integer string=w1218:string)  [unwired: 1 in]
        n278 = Fract/Exp String To Number(string=w1215) -> (number=w1191:dbl[])  [unwired: 3 in, 1 out]
        n279 = Concatenate Strings(w1203, "-vsu2-" ("Substring"), w1218, w1182, ".txt" ("Substring")) -> (w1216:string)
        n280 = String To Path(string=w1216) -> (path=w1207:path)
        n281 = Index Array(array=w1191, index=1 ("Index")) -> (element=w1190:dbl)
        n282 = Index Array(array=w1191, index=0 ("Index")) -> (element=w1188:dbl)
        n283 = call "4155C Config VSU2 Stress.vi"("error in (no error)"=w1220, "VSU2"=w1188, "Display on/off"=TRUE, "VISA session"=w1221) -> ("error out"=w1222:errorcluster, "dup VISA resource name"=w1223:refnum<visa-resource-name>)
        n284 = call "4155C Apply Stress.vi"("error in (no error)"=w1222, "Duration"=w1190, "Emergency Stop"=w1202, "VISA resource name in"=w1223) -> ("error out"=w1200:errorcluster, "VISA Resource Name out"=w1198:refnum<visa-resource-name>)
        n285 = VISA Write(VISA resource name=w1198, write buffer=":DISP ON" ("write buffer (\"\")"), error in (no error)=w1200) -> (VISA resource name out=w1197:refnum<visa-resource-name>, error out=w1199:errorcluster)  [unwired: 1 out]
        n286 = call <vilib>:"compatOverwrite.vi"("overwrite (F)"=TRUE) -> ("overwrite?"=w1187:T7)
        n287 = Open/Create/Replace File(file path (use dialog)=w1207, error in=w1199, operation (0:open)=w1187) -> (refnum out=w1210:refnum<file>, error out=w1209:errorcluster)  [unwired: 3 in, 1 out]
        n288 = call "4155C Write array to file.vi"("Byte Stream File Refnum"=w1210, "Header"=string[] ["VSU2 pulse completed successfully", ""], "error in (no error)"=w1209) -> ("dup refnum"=w1212:refnum<file>, "error out"=w1211:errorcluster)  [unwired: 2 in]
        n289 = Close File(refnum=w1212, error in=w1211) -> (error out=w1205:errorcluster)  [unwired: 1 out]
      }
      frame "sample-fpp" {
        w1243 = string[] ["Time /s", "Id VgVd /A", "Ig VgVd /A", "Vp1 VgVd /V", "Vp2 VgVd /V"] ("Header")
        w1247 = "%d" ("format string")
        n290 = Number To Decimal String(number=w1232) -> (decimal integer string=w1295:string)  [unwired: 1 in]
        n291 = Fract/Exp String To Number(string=w1292) -> (number=w1280:dbl[])  [unwired: 3 in, 1 out]
        n292 = Concatenate Strings(w1286, "-samplefpp-" ("Substring"), w1295, w1231, ".txt" ("Substring")) -> (w1293:string)
        n293 = String To Path(string=w1293) -> (path=w1255:path)
        n294 = Index Array(array=w1280, index=0 ("Index")) -> (element=w1241:dbl)
        n295 = Index Array(array=w1280, index=1 ("Index")) -> (element=w1240:dbl)
        n296 = Index Array(array=w1280, index=2 ("Index")) -> (element=w1288:dbl)
        n297 = Index Array(array=w1280, index=3 ("Index")) -> (element=w1278:dbl)
        n298 = call "4155C Config Sampling Measurements FPP.vi"("VISA session"=w1298, "Num Points"=w1288, "Vg"=w1241, "Display on/off"=TRUE, "Gate Compliance"=w1287, "Drain Compliance"=w1296, "Standby"="Standby", "error in (no error)"=w1297, "Timings"=w1285, "Vd"=w1240, "Sample time"=w1278) -> ("dup VISA resource name"=w1257:refnum<visa-resource-name>, "error out"=w1256:errorcluster)  [unwired: 3 in]
        n299 = Number To Decimal String(number=w1241) -> (decimal integer string=w1267:string)  [unwired: 1 in]
        n300 = call "4155C Take Sample FPP.vi"("VISA resource name in"=w1257, "error in (no error)"=w1256, "Emergency Stop"=w1258) -> ("Time"=w1262:dbl[], "Vp1"=w1272:dbl[], "VISA Resource Name out"=w1238:refnum<visa-resource-name>, "Ig"=w1260:dbl[], "Id"=w1261:dbl[], "Vp2"=w1270:dbl[], "error out"=w1259:errorcluster)  [unwired: 10 in]
        n301 = Insert Into Array(array=dbl[][] [] ("Input Array"), new element=w1262) -> (w1276:dbl[][])  [unwired: 2 in]
        n302 = Number To Decimal String(number=w1240) -> (decimal integer string=w1265:string)  [unwired: 1 in]
        n303 = Insert Into Array(array=w1276, new element=w1261) -> (w1275:dbl[][])  [unwired: 2 in]
        n304 = Concatenate Strings("(Vg = " ("Substring"), w1267, "V, Vd = " ("Substring"), w1265, "V)" ("Substring")) -> (w1263:string)
        n305 = Insert Into Array(array=w1275, new element=w1260) -> (w1274:dbl[][])  [unwired: 2 in]
        n306 = Insert Into Array(array=w1274, new element=w1272) -> (w1271:dbl[][])  [unwired: 2 in]
        n307 = Insert Into Array(array=w1271, new element=w1270) -> (w1239:dbl[][])  [unwired: 2 in]
        n308 = call <vilib>:"compatOverwrite.vi"("overwrite (F)"=TRUE) -> ("overwrite?"=w1236:T7)
        n309 = Open/Create/Replace File(file path (use dialog)=w1255, error in=w1259, operation (0:open)=w1236) -> (refnum out=w1252:refnum<file>, error out=w1253:errorcluster)  [unwired: 3 in, 1 out]
        n310 = Array To Spreadsheet String(array=w1243, 3:w1247) -> (spreadsheet string=w1249:string)  [unwired: 1 in]
        n311 = Transpose 2D Array(2D array=w1239) -> (transposed array=w1269:dbl[][])
        n312 = Search and Replace String(replace all?=TRUE ("replace all? (F)"), input string=w1249, search string="VgVd", replace string=w1263) -> (result string=w1245:string)  [unwired: 4 in, 3 out]
        n313 = Spreadsheet String To Array(format string=w1247, spreadsheet string=w1245, array type (2D Dbl)=w1243) -> (array=w1244:string[])  [unwired: 1 in]
        n314 = call "4155C Write array to file.vi"("Byte Stream File Refnum"=w1252, "Header"=w1244, "Data Array"=w1269, "error in (no error)"=w1253) -> ("dup refnum"=w1250:refnum<file>, "error out"=w1251:errorcluster)  [unwired: 1 in]
        n315 = Close File(refnum=w1250, error in=w1251) -> (error out=w1237:errorcluster)  [unwired: 1 out]
      }
      frame "resample-fpp" {
        w1320 = string[] ["Time /s", "Id VgVd /A", "Ig VgVd /A", "Vp1 VgVd /V", "Vp2 VgVd /V"] ("Header")
        w1324 = "%d" ("format string")
        n316 = Number To Decimal String(number=w1306) -> (decimal integer string=w1364:string)  [unwired: 1 in]
        n317 = Fract/Exp String To Number(string=w1361) -> (number=w1313:dbl[])  [unwired: 3 in, 1 out]
        n318 = Concatenate Strings(w1357, "-resamplefpp-" ("Substring"), w1364, w1307, ".txt" ("Substring")) -> (w1362:string)
        n319 = String To Path(string=w1362) -> (path=w1332:path)
        n320 = Index Array(array=w1313, index=0 ("Index")) -> (element=w1319:dbl)
        n321 = Index Array(array=w1313, index=1 ("Index")) -> (element=w1318:dbl)
        n322 = Number To Decimal String(number=w1319) -> (decimal integer string=w1342:string)  [unwired: 1 in]
        n323 = call "4155C Take Sample FPP.vi"("VISA resource name in"=w1315, "error in (no error)"=w1314, "Emergency Stop"=w1333) -> ("Time"=w1337:dbl[], "Vp1"=w1347:dbl[], "VISA Resource Name out"=w1317:refnum<visa-resource-name>, "Ig"=w1335:dbl[], "Id"=w1336:dbl[], "Vp2"=w1345:dbl[], "error out"=w1334:errorcluster)  [unwired: 10 in]
        n324 = Insert Into Array(array=dbl[][] [] ("Input Array"), new element=w1337) -> (w1351:dbl[][])  [unwired: 2 in]
        n325 = Number To Decimal String(number=w1318) -> (decimal integer string=w1340:string)  [unwired: 1 in]
        n326 = Insert Into Array(array=w1351, new element=w1336) -> (w1350:dbl[][])  [unwired: 2 in]
        n327 = Concatenate Strings("(Vg = " ("Substring"), w1342, "V, Vd = " ("Substring"), w1340, "V)" ("Substring")) -> (w1338:string)
        n328 = Insert Into Array(array=w1350, new element=w1335) -> (w1349:dbl[][])  [unwired: 2 in]
        n329 = Insert Into Array(array=w1349, new element=w1347) -> (w1346:dbl[][])  [unwired: 2 in]
        n330 = Insert Into Array(array=w1346, new element=w1345) -> (w1312:dbl[][])  [unwired: 2 in]
        n331 = call <vilib>:"compatOverwrite.vi"("overwrite (F)"=TRUE) -> ("overwrite?"=w1311:T7)
        n332 = Open/Create/Replace File(file path (use dialog)=w1332, error in=w1334, operation (0:open)=w1311) -> (refnum out=w1329:refnum<file>, error out=w1330:errorcluster)  [unwired: 3 in, 1 out]
        n333 = Array To Spreadsheet String(array=w1320, 3:w1324) -> (spreadsheet string=w1326:string)  [unwired: 1 in]
        n334 = Transpose 2D Array(2D array=w1312) -> (transposed array=w1344:dbl[][])
        n335 = Search and Replace String(replace all?=TRUE ("replace all? (F)"), input string=w1326, search string="VgVd", replace string=w1338) -> (result string=w1322:string)  [unwired: 4 in, 3 out]
        n336 = Spreadsheet String To Array(format string=w1324, spreadsheet string=w1322, array type (2D Dbl)=w1320) -> (array=w1321:string[])  [unwired: 1 in]
        n337 = call "4155C Write array to file.vi"("Byte Stream File Refnum"=w1329, "Header"=w1321, "Data Array"=w1344, "error in (no error)"=w1330) -> ("dup refnum"=w1327:refnum<file>, "error out"=w1328:errorcluster)  [unwired: 1 in]
        n338 = Close File(refnum=w1327, error in=w1328) -> (error out=w1316:errorcluster)  [unwired: 1 out]
      }
      frame "serial" {
        n339 = local read "Enable Termination\nChar (T)"() -> (w1381:bool)
        n340 = local read "Termination char\n(0xA = '\\n' = LF)\n(0xD = '\\r' = CR)"() -> (w1380:u8)
        n341 = Index Array(array=w1388, index=0 ("Index")) -> (element=w1387:string)
        n342 = local read "parity"() -> (w1371:u16)
        n343 = local read "Delay before read (ms)"() -> (w1382:u32)
        n344 = local read "byte count"() -> (w1379:u32)
        n345 = local read "Timeout (ms)"() -> (w1378:u32)
        n346 = local read "VISA resource name"() -> (w1375:refnum<visa-resource-name>)
        n347 = local read "baud rate"() -> (w1374:u32)
        n348 = local read "Serial End Mode for Reads"() -> (w1373:u16)
        n349 = local read "data bits"() -> (w1372:u16)
        n350 = local read "stop bits"() -> (w1377:u16)
        n351 = local read "flow control"() -> (w1376:u16)
        n352 = call "Serial write and read v0.5.vi"("Delay before read (ms)"=w1382, "Termination char\n(0xA = '\\n' = LF)\n(0xD = '\\r' = CR)"=w1380, "Enable Termination\nChar (T)"=w1381, "parity"=w1371, "stop bits"=w1377, "string to write"=w1387, "flow control"=w1376, "byte count"=w1379, "Serial Settings:Serial End Mode for Reads"=w1373, "Timeout (ms)"=w1378, "error in (no error)"=w1393, "VISA resource name"=w1375, "baud rate"=w1374, "data bits"=w1372) -> ("Serial port output"=w1383:string, "error out"=w1392:errorcluster)
        n353 = Build Array (concatenate)(w1383, w1384) -> (w1385:string[])
      }
      frame "pump" {
        # "Time array for valve position"
        # "Valve position"
        # "Time array for absolute plunger position"
        # "Absolute plunger position"
        # "Remove \"_\""
        # "Check if hard stop is pressed."
        # "Check if halt is pressed."
        # "Check if pump is idle. Else halt."
        n354 = local read "Hard stop pump"() -> (w1423:bool)
        n355 = local read "Halt pump"() -> (w1426:bool)
        n356 = local read "Enable Termination\nChar (T)"() -> (w1440:bool)
        n357 = local read "Termination char\n(0xA = '\\n' = LF)\n(0xD = '\\r' = CR)"() -> (w1439:u8)
        n358 = Index Array(array=w1444, index=0 ("Index")) -> (element=w1421:string)
        n359 = case shown="\"Initialization\"" w1419 {
          tunnel: w1421 -> [w1480 _ w1482 w1483 w1484 w1485 _ _ w1488 w1489 _]
          tunnel: [w1480 "/1H" w1482 w1483 w1484 w1485 "/1H" "/1H" w1488 w1489 "/1H"] -> w1420
          frame "No error", Default {
          }
          frame "Initialization" {
          }
          frame "Invalid command" {
          }
          frame "Invalid operand" {
          }
          frame "Device not initialized" {
          }
          frame "Internal failure" {
          }
          frame "Plunger overload" {
          }
          frame "Valve overload" {
          }
          frame "Plunger move not allowed" {
          }
          frame "A/D converter failure" {
          }
          frame "Command overflow" {
          }
        }
        n360 = case shown="True" w1426 {
          tunnel: [w1494 "/1H"] -> w1425
          tunnel: w1420 -> [w1494 _]
          frame False {
          }
          frame True {
            n361 = local write "Halt pump"(FALSE) -> ()
          }
        }
        n362 = case shown="True" w1423 {
          tunnel: [w1491 "/1T"] -> w1424
          tunnel: w1425 -> [w1491 _]
          frame False {
          }
          frame True {
            n363 = local write "Hard stop pump"(FALSE) -> ()
          }
        }
        n364 = local read "Serial End Mode for Reads"() -> (w1432:u16)
        n365 = local read "flow control"() -> (w1435:u16)
        n366 = local read "stop bits"() -> (w1436:u16)
        n367 = local read "parity"() -> (w1430:u16)
        n368 = local read "Delay before read (ms)"() -> (w1441:u32)
        n369 = local read "byte count"() -> (w1438:u32)
        n370 = local read "Timeout (ms)"() -> (w1437:u32)
        n371 = local read "VISA resource name"() -> (w1434:refnum<visa-resource-name>)
        n372 = local read "baud rate"() -> (w1433:u32)
        n373 = local read "data bits"() -> (w1431:u16)
        n374 = String Subset(string=w1415, offset (0)=1) -> (substring=w1413:string)  [unwired: 1 in]
        n375 = call "SPM Pump v0.5.vi"("Termination char\n(0xA = '\\n' = LF)\n(0xD = '\\r' = CR)"=w1439, "Enable Termination\nChar (T)"=w1440, "Timeout (ms)"=w1437, "Serial Settings:Serial End Mode for Reads"=w1432, "byte count"=w1438, "Delay before read (ms)"=w1441, "Time <input>"=w1418, "error in (no error)"=w1449, "Serial port input"=w1424, "VISA resource name"=w1434, "parity"=w1430, "baud rate"=w1433, "stop bits"=w1436, "data bits"=w1431, "flow control"=w1435, "Time units <input>"=w1413) -> ("Input command"=w1412:string, "Pump status"=w1408:string, "Valve position"=w1410:i32, "Absolute plunger position"=w1422:i32, "Serial port"=w1417:string, "error out"=w1448:errorcluster)  [unwired: 2 in, 4 out]
        n376 = case shown="\"?\"" w1412 {
          tunnel: [w1461 w1469 w1475] -> w1429
          tunnel: w1428 -> [w1461 w1468 w1475]
          tunnel: w1422 -> [_ w1467 _]
          tunnel: w1409 -> [w1460 w1466 w1476]
          tunnel: [w1460 w1466 w1478] -> w1411
          tunnel: w1410 -> [_ _ w1477]
          tunnel: w1407 -> [_ w1465 w1473]
          tunnel: w1406 -> [w1459 w1464 w1474]
          tunnel: [w1459 w1463 w1474] -> w1405
          tunnel: [w1458 w1462 w1472] -> w1404
          tunnel: w1403 -> [w1458 w1462 w1471]
          frame "Q", Default {
          }
          frame "?" {
            n377 = Build Array (concatenate)(w1468, w1467) -> (w1469:i32[])
            n378 = Build Array (concatenate)(w1464, w1465) -> (w1463:i32[])
            n379 = call "4155C Split array.vi"("X data in"=w1463, "Y1 data in"=w1469) -> ("Array of clusters"=w1470:cluster{"Y data in":dbl[], "X data in":dbl[]}[])  [unwired: 5 in, 1 out]
            n380 = local write "Absolute plunger position vs time"(w1470) -> ()
          }
          frame "?6" {
            n381 = Build Array (concatenate)(w1476, w1477) -> (w1478:i32[])
            n382 = Build Array (concatenate)(w1471, w1473) -> (w1472:i32[])
            n383 = call "4155C Split array.vi"("X data in"=w1472, "Y1 data in"=w1478) -> ("Array of clusters"=w1479:cluster{"Y data in":dbl[], "X data in":dbl[]}[])  [unwired: 5 in, 1 out]
            n384 = local write "Valve position vs time"(w1479) -> ()
          }
        }
        n385 = Build Array (concatenate)(w1416, w1417) -> (w1442:string[])
      }
    }
    n386 = Build Array(w79, w125, w120) -> (w124:dbl[][])
    n387 = Build Array(w59, "Id max /A" ("VAR2 Name"), "Id min /A" ("VAR2 Name")) -> (w130:string[])
    n388 = Transpose 2D Array(2D array=w124) -> (transposed array=w123:dbl[][])
    n389 = Concatenate Strings(w56, "Prefix (Idmax-Idmin)", "Suffix (Idmax-Idmin)") -> (w137:string)
    n390 = Array To Spreadsheet String(array=w130, 3:"" ("format string")) -> (spreadsheet string=w129:string)  [unwired: 1 in]
    n391 = Array To Spreadsheet String(array=w123, 3:"%e" ("format string")) -> (spreadsheet string=w128:string)  [unwired: 1 in]
    n392 = String To Path(string=w137) -> (path=w136:path)
    n393 = Build Array(w129, w128) -> (w127:string[])
    n394 = Write to Text File(file (use dialog)=w136, text=w127, error in=w75) -> (refnum out=w138:refnum<file>, error out=w126:errorcluster)  [unwired: 1 in, 1 out]
    n395 = Close File(refnum=w138, error in=w126) -> (error out=w55:errorcluster)  [unwired: 1 out]
    n396 = Build Array(w51, w80) -> (w87:i32[][])
    n397 = Build Array(w59, "Absolute plunger position" ("VAR2 Name")) -> (w90:string[])
    n398 = Transpose 2D Array(2D array=w87) -> (transposed array=w78:i32[][])
    n399 = Array To Spreadsheet String(array=w90, 3:"" ("format string")) -> (spreadsheet string=w89:string)  [unwired: 1 in]
    n400 = Array To Spreadsheet String(array=w78, 3:"%e" ("format string")) -> (spreadsheet string=w86:string)  [unwired: 1 in]
    n401 = Build Array(w89, w86) -> (w92:string[])
    n402 = Concatenate Strings(w56, "Prefix (plunger)", "Suffix (plunger)") -> (w84:string)
    n403 = String To Path(string=w84) -> (path=w81:path)
    n404 = Write to Text File(file (use dialog)=w81, text=w92, error in=w55) -> (refnum out=w85:refnum<file>, error out=w94:errorcluster)  [unwired: 1 in, 1 out]
    n405 = Close File(refnum=w85, error in=w94) -> (error out=w54:errorcluster)  [unwired: 1 out]
    n406 = Concatenate Strings(w56, "Prefix (serial port log)", ".txt" ("Suffix")) -> (w102:string)
    n407 = Array To Spreadsheet String(array=w103, 3:"" ("format string")) -> (spreadsheet string=w108:string)  [unwired: 1 in]
    n408 = String To Path(string=w102) -> (path=w99:path)
    n409 = local write "Serial port data"(w108) -> ()
    n410 = Write to Text File(file (use dialog)=w99, text=w103, error in=w54) -> (refnum out=w104:refnum<file>, error out=w105:errorcluster)  [unwired: 1 in, 1 out]
    n411 = Close File(refnum=w104, error in=w105) -> (error out=w53:errorcluster)  [unwired: 1 out]
    n412 = Build Array(w50, w58) -> (w67:i32[][])
    n413 = Build Array(w59, "Valve position" ("VAR2 Name")) -> (w70:string[])
    n414 = Transpose 2D Array(2D array=w67) -> (transposed array=w60:i32[][])
    n415 = Array To Spreadsheet String(array=w70, 3:"" ("format string")) -> (spreadsheet string=w69:string)  [unwired: 1 in]
    n416 = Array To Spreadsheet String(array=w60, 3:"%e" ("format string")) -> (spreadsheet string=w66:string)  [unwired: 1 in]
    n417 = Build Array(w69, w66) -> (w72:string[])
    n418 = Concatenate Strings(w56, "Prefix (valve)", "Suffix (valve)") -> (w64:string)
    n419 = String To Path(string=w64) -> (path=w61:path)
    n420 = Write to Text File(file (use dialog)=w61, text=w72, error in=w53) -> (refnum out=w65:refnum<file>, error out=w74:errorcluster)  [unwired: 1 in, 1 out]
    n421 = Close File(refnum=w65, error in=w74) -> (error out=w52:errorcluster)  [unwired: 1 out]
  }
  "error out" <- w9
